vi "Multi_Run_Prog.vi"(0 "Command filename":path, 1 "Mode":T9(ring), 2 "Table":T6[](array[typedef]) {"Carrier_2 Q (l/min)" format="%#.2f"; "Row Duration (mins)" format="%#.1f"; "Row No" min=0; "Trace Gas Concentration (%)" min=0.0 format="%#_4f"; "Carrier_1 Q (l/min)" format="%#.4f"; "Start X" format="%#.2f"; "Start Y" format="%#.2f"; "Start Z" format="%#.2f"; "End X" format="%#.2f"; "End Y" format="%#.2f"; "End Z" format="%#.2f"; "Tunnel Speed" format="%#.2f"; "Averaging time (mins)" min=0.0 format="%#.2f"}, 3 "Work in Tunnel Coordinates?":T1) -> (17 "Status":T2)   [LabVIEW 2022 SP3]
uses:
  Anemometry Sub Vis/Gen Trav/Traverse_cluster.ctl
  Anemometry Sub Vis/Gen Trav/Spacing.ctl
  Anemometry Sub Vis/Controls/Multi_run_mode.ctl
  Anemometry Sub Vis/Gen Trav/Route mapping/Route_Display_Mode.ctl
  Anemometry Sub Vis/Controls/User_Specific_mode.ctl
  Anemometry Sub Vis/Controls/Multi_Run_Case.ctl
  Anemometry Sub Vis/Gen Trav/Multi_Run_Status.ctl
  Anemometry Sub Vis/Controls/Tunnel_Coordinates.ctl
  Anemometry Sub Vis/Controls/Post_Process.ctl
  ADAM Client/Sub VIs/ADAM Controls/Traverse_Level_State.ctl
  Anemometry Sub Vis/Controls/PP Raw data file cluster.ctl
  ADAM Client/Sub VIs/ADAM Controls/Tunnel_speed_mode.ctl
  Anemometry Sub Vis/Controls/Overhead.ctl
  ADAM Client/Sub VIs/ADAM Controls/Remember_value_mode.ctl
  Anemometry Sub Vis/Gen Trav/Trav_mode.ctl
  Anemometry Sub Vis/Controls/Home.ctl
  ADAM Client/Sub VIs/ADAM Controls/Quick_local_ADAM_Table.ctl
  ADAM Client/Sub VIs/ADAM Controls/Client_Source_Status.ctl
  ADAM Client/Sub VIs/ADAM Controls/Update_scan_value.ctl
  <vilib>/Utility/error.llb/Trim Whitespace One-Sided.vi
  Anemometry Sub Vis/Globals/Meas_global.vi
  Anemometry Sub Vis/Globals/Trav_pos_global.vi
  Anemometry Sub Vis/Globals/Preference_global.vi
  Anemometry Sub Vis/Globals/Extra_Commands_Global.vi
  Anemometry Sub Vis/Gen Trav/Route mapping/Route_mapping_global.vi
  ADAM Serial/Instrument drivers/Traverses/~subVIs/DriveConfigGlobal.vi
  Anemometry Sub Vis/Globals/Gas_management_global.vi
  <vilib>/Utility/config.llb/Write Key (Double).vi
  <vilib>/Utility/config.llb/NI_LVConfig.lvlib
panel:
  out "remainingTime":string
  out "Progress":i32(slide) scale=0.0..1.0
  out "PredictedEnd":timestamp format="%<%H:%M\n%a %d>T"
  out "StartTime":timestamp format="%<%H:%M\n%a %d>T"
  in  "Fast Plotting?":bool
  in  "Sort Single\nMeasurements":bool
  out "Last Row Run":i32
  in  "Stop after Repeats":bool
  out "Overhead Factor":dbl format="%.3f"
  out "Estimated Completion":string
  out "Max Tunnel Speed":dbl format="%.2f"
  out "Pause message":string
  in  "Pause":bool
  out "Non Starter":bool
  out "No of Rows":i32
  in  "Synchronization Start No":i32=1 min=1 max=100
  out "Case":T3
  out "Simulate/Run":T4
  in  "Display Mode":T5=enum."Display View on Crash"
  in  "stop":bool
  out "Current Row":i32
  # "X           Y          Z"
  # "Start"
  # "End"
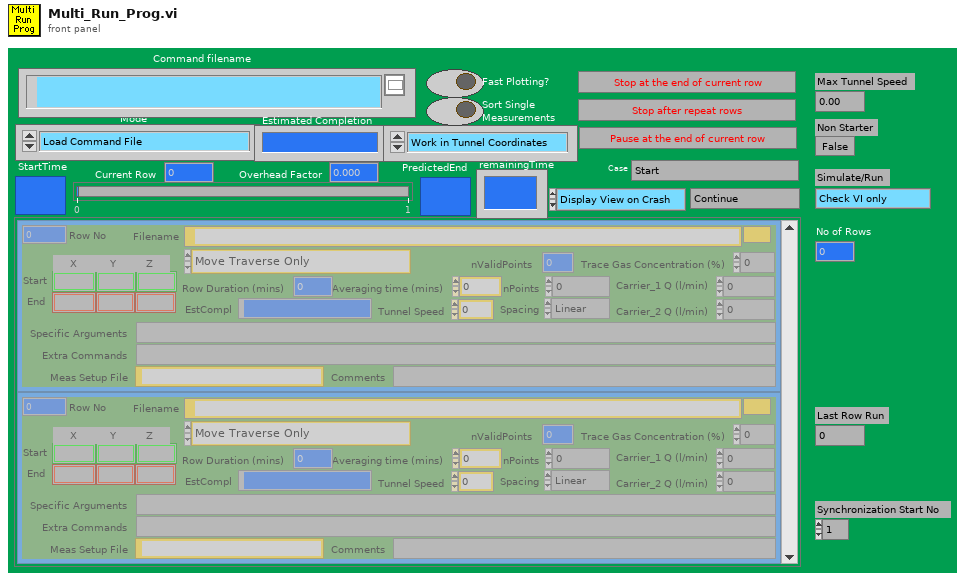
[diagram p1: front panel]
types:
  T1 = typedef "Tunnel_Coordinates.ctl" = enum16{"Work in Tunnel Coordinates", "Work in Model Coordinates"}
  T2 = typedef "Multi_Run_Status.ctl" = enum16{"Continue", "Continue with Error", "Jump to Next Point", "Jump to Next Row", "Jump To Fall Back", "Terminate Run"}
  T3 = typedef "Multi_Run_Case.ctl" = enum16{"Start", "Load Setup From File", "Has file been edited in Excel?", "Check Max Tunnel Speed", "Pre Check Row", "Check Rows", "Remove blank end rows", "Do results files already exist?", "More Multi Run Checks", "First Save Setup file", "Setup Route checking", "Initialise Measurement Prog", "Input Current Position", "Experimental setup control", "Check source flowrates", "Setup for running mode", "Skip Blank Rows", "Which row to execute next", "Evaluate IF Statement", "Perform Measurement Setup", "Set Measurement Conditions", "Execute Row", "Calculate Row TIme", "Update time estimate", "Pause Multi Run Program", "Do Another Row?", "Find Next Fall Back Row", "Shut down source etc", "Email results to users", "Save run efficiency", "Remove Skipped Commands", "Show jumped positions", "Save Setup to File", "End"}
  T4 = typedef "User_Specific_mode.ctl" = enum16{"Check VI only", "Run VI"}
  T5 = typedef "Route_Display_Mode.ctl" = enum16{"Display View Always", "Display View on Crash"}
  T6 = typedef "Traverse_cluster.ctl" = cluster{"Start X":sgl, "Start Y":sgl, "Start Z":sgl, "End X":sgl, "End Y":sgl, "End Z":sgl, "nPoints":i32, "Spacing":T7, "Filename":path, "Tunnel Speed":dbl, "Averaging time (mins)":dbl, "Extra Commands":string, "Carrier_1 Q (l/min)":dbl, "Carrier_2 Q (l/min)":dbl, "Trace Gas Concentration (%)":dbl, "Specific Arguments":string, "Comments":string, "Row No":i32, "Row Type Selector":T8, "EstCompl":string, "Row Duration (mins)":dbl, "nValidPoints":i32, "Meas Setup File":string}
  T7 = typedef "Spacing.ctl" = enum16{"Linear", "Log", "Gauss", "Specified", "N/A"}
  T8 = typedef "Multi_run_mode.ctl" = enum16{"Move Traverse Only", "Set Tunnel Speed Only", "Set Source Only", "Set Measurement Conditions", "Single Measurement", "Vertical Profile", "Lateral Profile", "Longitudinal Profile", "Multi-Axis Profile", "Explore Volume", "Auto Calibrate", "Meas Fast FID Bkgnd", "Check Beam Power", "Scanning Valve Measurement", "Run VI Named:", "Set ADAM Ch", "Wait (minutes)", "Send Message", "Synchronize With:", "Fall Back to this Row", "Turn Off Row Repeating", "Traverse 3D Volume", "Blank Row", "Jump to Fall Back Row"}
  T9 = enum16{"Load Command File", "Save Command File", "Check Multi Run Prog", "Check Multi Run Prog With Live Moves", "Run Multi Run Prog"}
  T10 = typedef "Post_Process.ctl" = enum16{"Take New Data", "Post Process Raw Data File"}
  T11 = typedef "PP Raw data file cluster.ctl" = cluster{"Raw Data File":path, "Results File":path}
  T12 = typedef "Traverse_Level_State.ctl" = enum16{"Running", "Complete"}
  T13 = enum32{"existing file", "new file", "new or existing file", "existing dir", "new dir", "new or existing dir", "existing file (use LLBs)", "new file (use LLBs)", "new or existing file (use LLBs)", "new or existing file or directory (use LLBs)"}
  T14 = typedef "Tunnel_speed_mode.ctl" = enum16{"Set Speed", "Set Speed then wait", "Is tunnel speed allowable?"}
  T15 = enum16{"All Channel Names", "Valid Channel Names"}
  T16 = typedef "Overhead.ctl" = enum16{"Update total times", "Read Current Overhead", "Re Scale totals to 3 hrs", "Initialise totals to 3hr"}
  T17 = typedef "Remember_value_mode.ctl" = enum16{"Read only", "Read and Write"}
  T18 = typedef "Home.ctl" = enum16{"Don't Home", "Home  +X", "Home  -X", "Home  +Y", "Home  -Y", "Home  +Z", "Home  -Z"}
  T19 = typedef "Trav_mode.ctl" = enum16{"Move traverse", "Read traverse position", "Teach Position"}
  T20 = typedef "Quick_local_ADAM_Table.ctl" = enum16{"Read Global", "Load Global From ADAM Table", "Write Global"}
  T21 = typedef "Client_Source_Status.ctl" = enum16{"Not Using", "Using", "Must Have"}
  T22 = typedef "Update_scan_value.ctl" = cluster{"Channel Name":string, "New Value":dbl, "!Auto_Off":bool}
  T23 = typedef "DriveProperties.ctl" = cluster{"Channel Name":string, "Vel. Default":sgl, "Acc. Default":sgl, "Vel. Max":sgl, "Vel. Min":sgl, "Acc. Max":sgl, "Acc. Min":sgl, "Pulses/unit":sgl, "Address":u8, "Pulse Offset":i32, "Pos Tolerance":sgl, "Pulses/rev":sgl, "Backlash/Eng units":sgl, "Current Pos":sgl, "Ch Status":enum16{"Active", "Offline", "Simulate"}, "Port Name":string, "Axis Transform mode":string, "Metadata Ch Name":string, "Type":T24, "De Power Motor":enum16{"TRUE", "FALSE"}, "ConfigString":string}
  T24 = typedef "Traverse Type.ctl" = enum16{"MCode", "Dynamixel"}
  T25 = typedef "GMU Gas Line Name.ctl" = enum16{"GMU1 Source", "GMU2 Source", "GMU2 Calib", "CPP GRC-A", "CPP GRC-B"}
  T26 = typedef "Status_Cluster.ctl" = cluster{"Status":T2, "Error Type":string, "Error Description":string}
  T27 = typedef "Server_Comms.ctl" = enum16{"Do Not Link To Server", "Server Link Healthy"}
  T28 = typedef "NI_LVConfig.lvlib/Config Data RefNum.ctl" = refnum<k1>
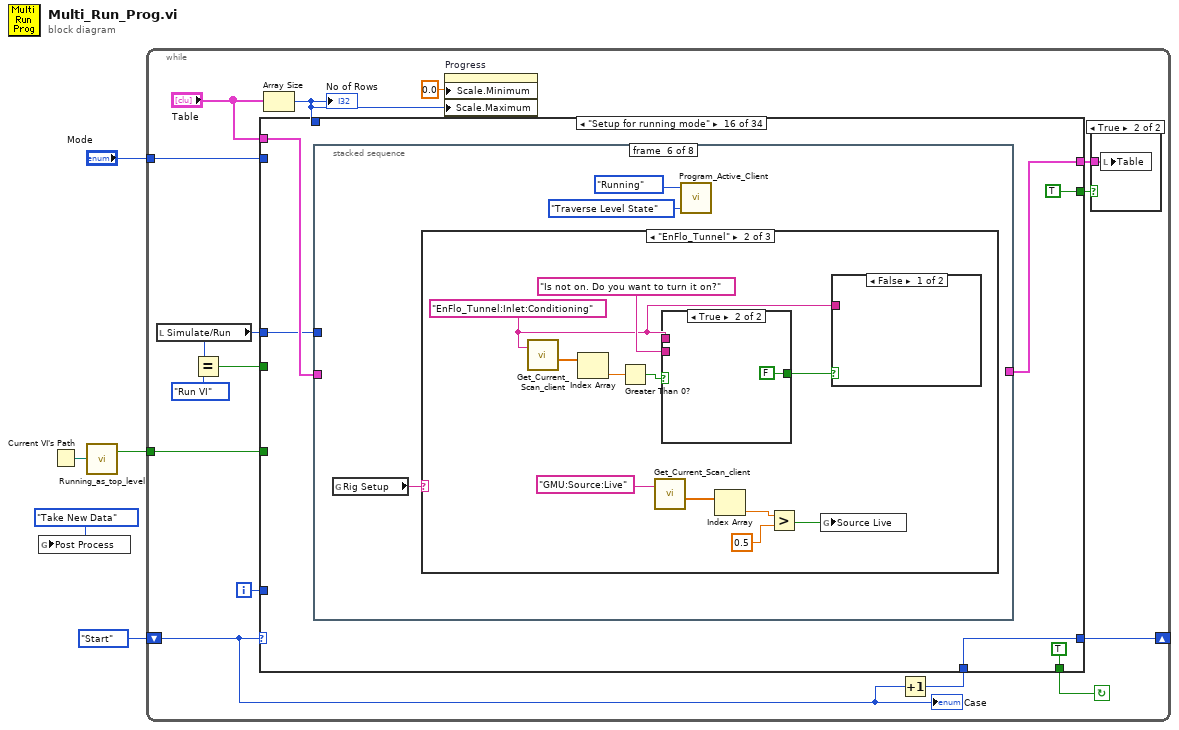
[diagram p0: block diagram]
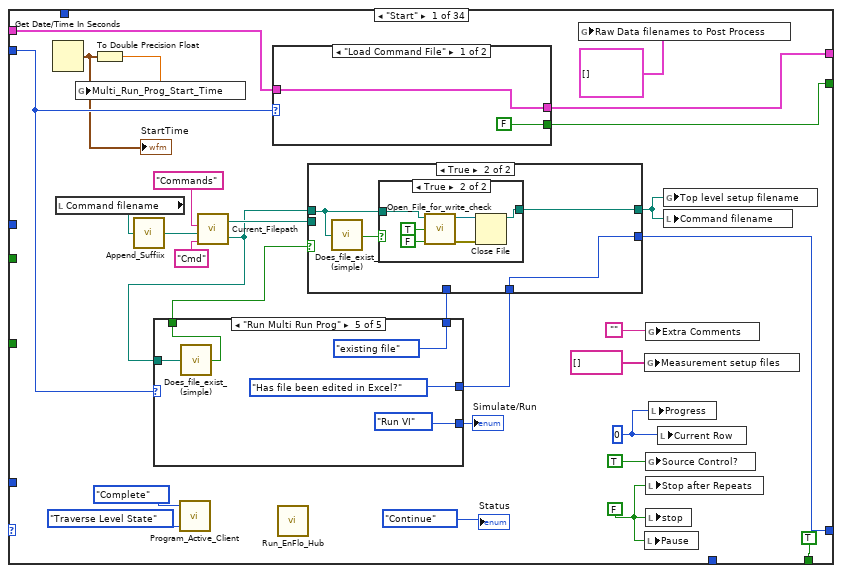
[diagram p3: hidden frame]
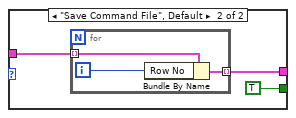
[diagram p4: hidden frame]
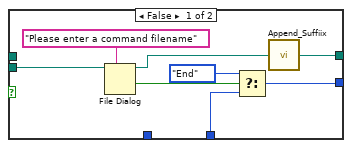
[diagram p5: hidden frame]
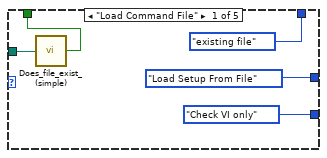
[diagram p7: hidden frame]
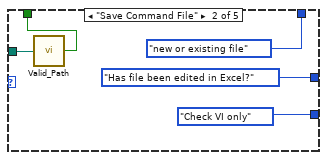
[diagram p8: hidden frame]
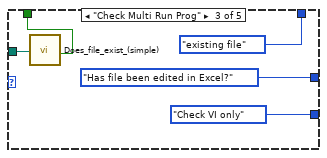
[diagram p9: hidden frame]
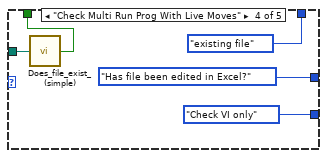
[diagram p10: hidden frame]
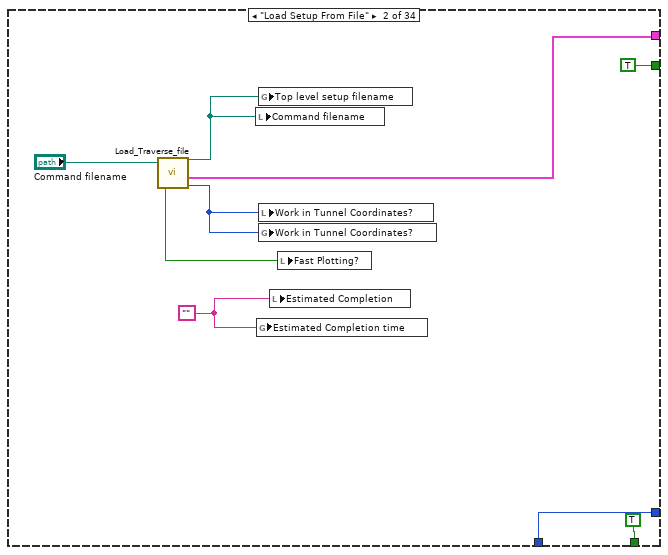
[diagram p11: hidden frame]
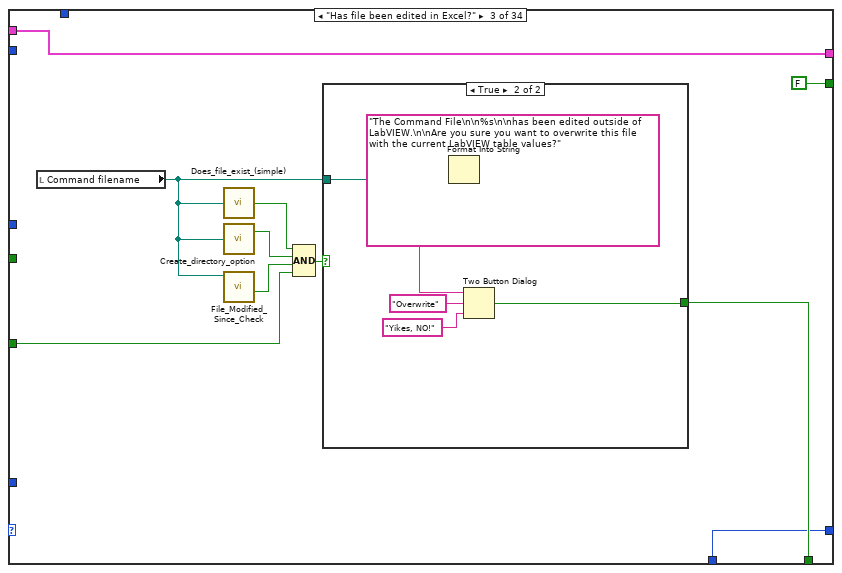
[diagram p12: hidden frame]
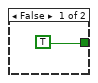
[diagram p13: hidden frame]
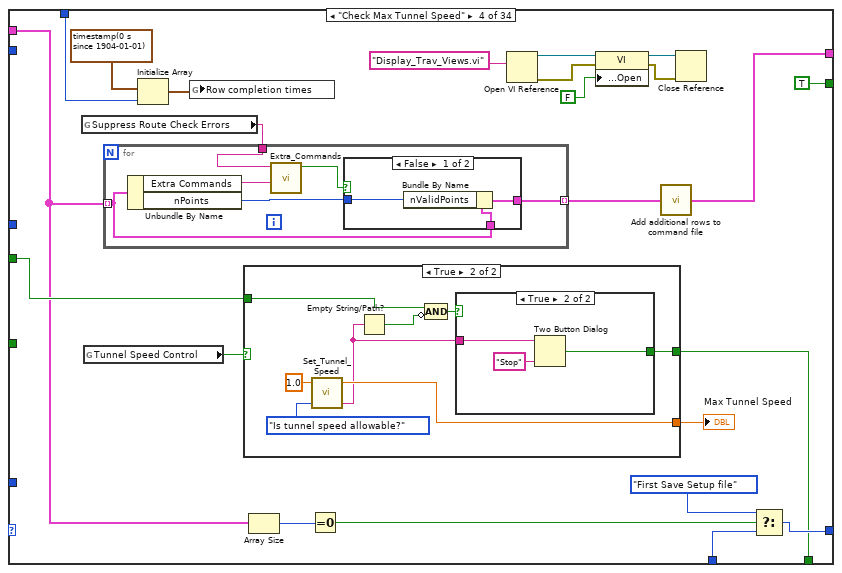
[diagram p14: hidden frame]
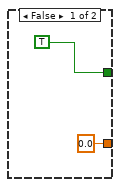
[diagram p16: hidden frame]
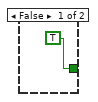
[diagram p17: hidden frame]
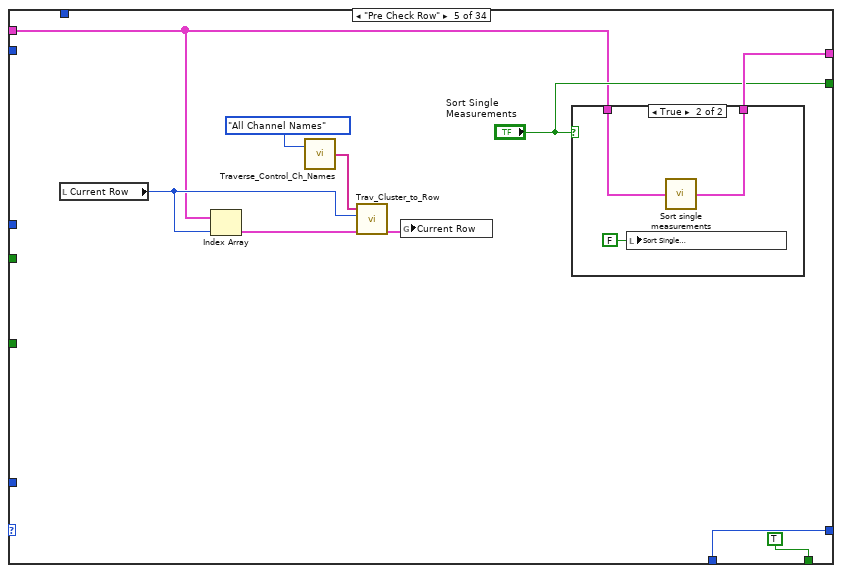
[diagram p18: hidden frame]
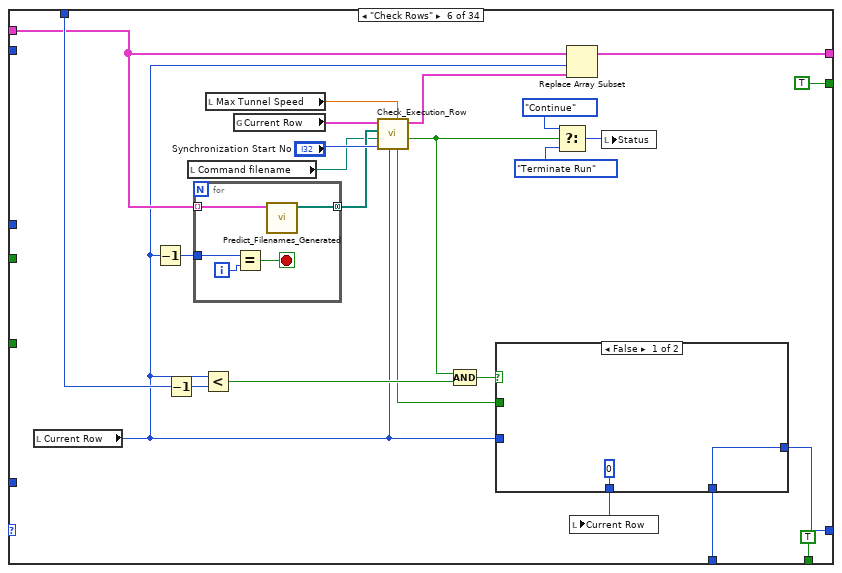
[diagram p20: hidden frame]
diagram:
  n1 = global write "Meas_global.vi" "Post Process"(Post_Process."Take New Data" ("Post Process")) -> ()
  n2 = Current VI's Path() -> (path=w2:path)
  n3 = call "Running_as_top_level.vi"("Vi path name"=w2) -> ("Top Level"=w1:bool)  [unwired: 1 out]
  n4 = while {
    shift-left: Multi_Run_Case."Start" ("Multi Run Case") -> [w17]
    shift-right: [w14] -> _
    tunnel: "Mode" -> [w20]
    tunnel: w1 -> [w9]
    i -> [w18]
    stop <- w8 continue-if-true
    n5 = local read "Simulate/Run"() -> (w11:T4)
    n6 = Equal?(x=w11, y=User_Specific_mode."Run VI" ("Simulate/Run")) -> (x = y?=w10:bool)
    n7 = Array Size(array="Table") -> (size(s)=w7:i32)
    "No of Rows" <- w7
    n8 = property on="Progress" class="Slide (strict)"("Scale.Minimum"=0.0 ("Scale.Range:Minimum"), "Scale.Maximum"=w7) -> ()  [unwired: 2 in, 2 out]
    n9 = Increment(x=w17) -> (x+1=w19:T3)
    n10 = case shown="\"Setup for running mode\"" w17 {
      tunnel: [TRUE TRUE w118 w134 TRUE TRUE TRUE TRUE TRUE TRUE TRUE ("Continue?") TRUE ("Continue?") TRUE TRUE TRUE TRUE ("Continue?") TRUE ("Continue?") TRUE ("Continue?") TRUE TRUE ("Continue?") TRUE TRUE TRUE TRUE TRUE TRUE TRUE TRUE TRUE TRUE TRUE TRUE TRUE FALSE] -> w8
      tunnel: w20 -> [w37 _ _ _ _ _ _ _ _ w539 _ _ _ _ _ _ _ _ _ _ _ _ _ _ _ _ _ _ _ _ _ _ w1456 _]
      tunnel: "Table" -> [w47 _ w115 w132 w175 w193 w232 w256 w413 w541 w564 w627 w645 w652 w660 w677 w766 w814 w935 w985 w998 w1089 w1128 w1160 w1203 w1247 w1289 w1334 w1366 w1414 w1425 w1443 w1475 w1525]
      tunnel: w11 -> [_ _ _ _ _ _ _ w255 _ _ _ _ _ _ w659 w676 _ w812 _ w982 w995 w1088 _ w1157 _ w1253 _ _ _ _ _ _ w1466 _]
      tunnel: w19 -> [_ w107 w117 w147 w183 w199 w243 w259 w412 w538 w567 w625 w646 w651 w664 w679 w768 w810 w940 w986 w1005 w1086 w1121 w1162 w1206 _ _ w1320 w1368 w1416 w1428 w1446 w1473 w1524]
      tunnel: w18 -> [_ _ _ _ _ _ _ _ _ _ _ _ _ _ _ _ _ _ _ _ _ _ _ _ w1204 _ _ _ _ _ _ _ _ _]
      tunnel: [w45 w107 w117 w146 w183 w198 w243 w259 w412 w534 w567 w624 w646 w651 w662 w679 w768 w811 w939 w986 w1006 w1086 w1121 w1162 w1207 w1242 w1296 w1329 w1368 w1416 w1428 w1446 w1473 w1524] -> w14
      tunnel: [w36 TRUE FALSE ("Rows Added ?") TRUE ("Rows Added ?") "Sort Single\nMeasurements" TRUE TRUE FALSE FALSE TRUE FALSE FALSE FALSE FALSE FALSE TRUE FALSE ("Rows Added ?") FALSE ("Rows Added ?") FALSE FALSE ("Rows Added ?") FALSE FALSE FALSE TRUE ("Rows Added ?") FALSE FALSE FALSE FALSE FALSE FALSE TRUE TRUE TRUE FALSE] -> w15
      tunnel: w7 -> [_ _ _ w141 _ w203 w234 _ _ _ _ _ _ _ _ _ w769 w813 _ _ _ _ _ w1156 _ w1245 w1291 _ _ _ _ _ w1452 _]
      tunnel: [w46 w108 w115 w129 w177 w206 w238 w256 w413 w542 w564 w627 w645 w652 w660 w675 w766 w815 w935 w985 w998 w1089 w1128 w1159 w1203 w1247 w1289 w1334 w1366 w1414 w1424 w1443 w1474 w1525] -> w13
      tunnel: w10 -> [_ _ _ w133 _ _ _ _ _ _ _ _ _ w649 w658 _ _ _ w929 _ _ _ w1120 _ _ _ _ _ _ _ _ _ _ _]
      tunnel: w9 -> [_ _ w114 _ _ _ _ w254 _ _ _ _ _ _ _ _ _ _ _ _ _ _ _ _ _ _ _ _ _ _ _ _ _ _]
      frame "Start" {
        w34 = FALSE ("Measurment setup Found?")
        w22 = 0 ("Currently on Row")
        n11 = Get Date/Time In Seconds() -> (seconds since 1Jan1904=w23:timestamp)
        "StartTime" <- w23
        n12 = local read "Command filename"() -> (w39:path)
        n13 = To Double Precision Float(number=w23) -> (double precision float=w25:dbl)
        n14 = global write "Trav_pos_global.vi" "Multi_Run_Prog_Start_Time"(w25) -> ()
        n15 = call "Append_Suffiix.vi"("Results file"=w39) -> ("appended path"=w30:path)
        n16 = call "Program_Active_Client.vi"("Mode"=enum16{"Program Active", "Traverse Level State"}."Traverse Level State", "Traverse level State"=Traverse_Level_State."Complete") -> ()  [unwired: 1 in, 3 out]
        n17 = call "Current_Filepath.vi"("Short_Name"="Cmd" ("Data Type"), "Filename in"=w30, "Data Type"="Commands") -> ("Filename Out"=w27:path, "Directory"=w29:path)  [unwired: 1 in]
        n18 = case shown="\"Run Multi Run Prog\"" w37 {
          tunnel: [User_Specific_mode."Check VI only" ("Simulate/Run") User_Specific_mode."Check VI only" ("Simulate/Run") User_Specific_mode."Check VI only" ("Simulate/Run") User_Specific_mode."Check VI only" ("Simulate/Run") User_Specific_mode."Run VI" ("Simulate/Run")] -> w48
          tunnel: [Multi_Run_Case."Load Setup From File" ("Multi Run Case") Multi_Run_Case."Has file been edited in Excel?" ("Multi Run Case") Multi_Run_Case."Has file been edited in Excel?" ("Multi Run Case") Multi_Run_Case."Has file been edited in Excel?" ("Multi Run Case") Multi_Run_Case."Has file been edited in Excel?" ("Multi Run Case")] -> w44
          tunnel: [T13."existing file" ("select mode (2)") T13."new or existing file" ("select mode (2)") T13."existing file" ("select mode (2)") T13."existing file" ("select mode (2)") T13."existing file" ("select mode (2)")] -> w35
          tunnel: w27 -> [w78 w83 w87 w93 w98]
          tunnel: [w77 w82 w88 w92 w97] -> w26
          frame "Load Command File" {
            n19 = call "Does_file_exist_(simple).vi"("Pathname"=w78) -> ("exists?"=w77:bool)
          }
          frame "Save Command File" {
            n20 = call "Valid_Path.vi"("Filename"=w83) -> ("Valid Path?"=w82:bool)
          }
          frame "Check Multi Run Prog" {
            n21 = call "Does_file_exist_(simple).vi"("Pathname"=w87) -> ("exists?"=w88:bool)
          }
          frame "Check Multi Run Prog With Live Moves" {
            n22 = call "Does_file_exist_(simple).vi"("Pathname"=w93) -> ("exists?"=w92:bool)
          }
          frame "Run Multi Run Prog" {
            n23 = call "Does_file_exist_(simple).vi"("Pathname"=w98) -> ("exists?"=w97:bool)
          }
        }
        "Simulate/Run" <- w48
        n24 = case shown="\"Load Command File\"" w37 {
          tunnel: w47 -> [w51 w54]
          tunnel: [w51 w53] -> w46
          tunnel: [FALSE TRUE] -> w36
          frame "Load Command File" {
          }
          frame "Save Command File", Default {
            n25 = for {
              tunnel: w54 -> [w57] mode=indexing
              tunnel: [w56] -> w53 mode=indexing
              i -> [w55]
              n26 = Bundle By Name(cluster=w57, "Row No"=w55) -> (w56:T6)
            }
          }
        }
        n27 = call "Run_EnFlo_Hub.vi"() -> ()  [unwired: 1 in, 7 out]
        n28 = case shown="True" w26 {
          tunnel: [w63 w69] -> w45
          tunnel: w44 -> [w64 w69]
          tunnel: w27 -> [_ w67]
          tunnel: [w62 w68] -> w38
          tunnel: w35 -> [_ _]
          tunnel: w29 -> [w58 _]
          frame False {
            n29 = File Dialog(7:"Please enter a command filename" ("prompt"), 11:w58) -> (1:w60:bool, 3:w61:path)  [unwired: 1 in, 6 out]
            n30 = Select(t=Multi_Run_Case."End" ("Multi Run Case"), s=w60, f=w64) -> (s? t:f=w63:T3)
            n31 = call "Append_Suffiix.vi"("Results file"=w61) -> ("appended path"=w62:path)
          }
          frame True {
            n32 = call "Does_file_exist_(simple).vi"("Pathname"=w67) -> ("exists?"=w66:bool)
            n33 = case shown="True" w66 {
              tunnel: [w70 w72] -> w68
              tunnel: w67 -> [w70 w71]
              frame False {
              }
              frame True {
                n34 = call "Open_File_for_write_check.vi"("advisory dialog? (display:T)"=FALSE, "append to file? (new file:F)"=TRUE, "file path"=w71) -> ("error out"=w74:errorcluster, "refnum"=w73:refnum<file>)  [unwired: 7 out]
                n35 = Close File(refnum=w73, error in=w74) -> (path=w72:path)  [unwired: 1 out]
              }
            }
          }
        }
        n36 = global write "Trav_pos_global.vi" "Raw Data filenames to Post Process"(T11[] [] ("Raw Data filenames to Post Process")) -> ()
        n37 = global write "Trav_pos_global.vi" "Measurement setup files"(string[] [] ("Measurement setup files")) -> ()
        n38 = local write "Pause"(w34) -> ()
        n39 = global write "Meas_global.vi" "Extra Comments"("") -> ()
        n40 = global write "Trav_pos_global.vi" "Source Control?"(TRUE ("Source Control?")) -> ()
        n41 = local write "Stop after Repeats"(w34) -> ()
        n42 = local write "stop"(w34) -> ()
        n43 = local write "Progress"(w22) -> ()
        n44 = local write "Current Row"(w22) -> ()
        n45 = global write "Trav_pos_global.vi" "Top level setup filename"(w38) -> ()
        n46 = local write "Command filename"(w38) -> ()
        "Status" <- Multi_Run_Status."Continue" ("Status")
      }
      frame "Load Setup From File" {
        w103 = ""
        n47 = call "Load_Traverse_file.vi"("Setup filename"="Command filename") -> ("Fast Plotting?"=w102:bool, "Setup filename Out"=w105:path, "Table"=w108:T6[], "Work in Tunnel Coordinates?"=w104:T1)  [unwired: 2 out]
        n48 = local write "Command filename"(w105) -> ()
        n49 = global write "Trav_pos_global.vi" "Estimated Completion time"(w103) -> ()
        n50 = global write "Trav_pos_global.vi" "Top level setup filename"(w105) -> ()
        n51 = local write "Work in Tunnel Coordinates?"(w104) -> ()
        n52 = global write "Trav_pos_global.vi" "Work in Tunnel Coordinates?"(w104) -> ()
        n53 = local write "Estimated Completion"(w103) -> ()
        n54 = local write "Fast Plotting?"(w102) -> ()
      }
      frame "Has file been edited in Excel?" {
        n55 = local read "Command filename"() -> (w112:path)
        n56 = call "Does_file_exist_(simple).vi"("Pathname"=w112) -> ("exists?"=w113:bool)
        n57 = call "Create_directory_option.vi"("Filename"=w112) -> ("Path is to existing File"=w119:bool)  [unwired: 1 out]
        n58 = call "File_Modified_Since_Check.vi"("File Path"=w112) -> ("modifiedSinceRead"=w111:bool)  [unwired: 7 in, 1 out]
        n59 = Compound Arithmetic op=AND(w113, w119, w111, w114) -> (w120:bool)
        n60 = case shown="True" w120 {
          tunnel: w112 -> [_ w127]
          tunnel: [TRUE ("T button?") w122] -> w118
          frame False {
          }
          frame True {
            n61 = Format Into String(format string="The Command File\n\n%s\n\nhas been edited outside of LabVIEW.\n\nAre you sure you want to overwrite this file with the current LabVIEW table values?" ("Format String"), w127) -> (resulting string=w125:string)  [unwired: 2 in, 1 out]
            n62 = Two Button Dialog(message=w125, 1:"Yikes, NO!" ("F button name (\"Cancel\")"), 2:"Overwrite" ("T button name (\"OK\")")) -> (T button?=w122:bool)
          }
        }
      }
      frame "Check Max Tunnel Speed" {
        n63 = global read "Extra_Commands_Global.vi" "Suppress Route Check Errors"() -> (w128:string)
        n64 = global read "Preference_global.vi" "Tunnel Speed Control"() -> (w131:bool)
        n65 = for {
          tunnel: w132 -> [w155] mode=indexing
          tunnel: [w154] -> w130 mode=indexing
          tunnel: w128 -> [w152]
          n66 = Unbundle By Name(w155) -> ("Extra Commands"=w153:string, "nPoints"=w156:i32)
          n67 = call "Extra_Commands.vi"("String to Search"=w153, "Command"=w152) -> ("Command Found"=w151:bool)  [unwired: 1 in, 4 out]
          n68 = case shown="False" w151 {
            tunnel: w156 -> [w159 _]
            tunnel: w155 -> [w158 w160]
            tunnel: [w157 w160] -> w154
            frame False {
              n69 = Bundle By Name(cluster=w158, "nValidPoints"=w159) -> (w157:T6)
            }
            frame True {
            }
          }
        }
        n70 = Initialize Array(timestamp(0 s since 1904-01-01) ("seconds since 1Jan1904"), w141) -> (w142:timestamp[])
        n71 = global write "Trav_pos_global.vi" "Row completion times"(w142) -> ()
        n72 = case shown="True" w131 {
          tunnel: [0.0 ("Max allowable Tunnel Velocity") w169] -> w150
          tunnel: [TRUE w166] -> w134
          tunnel: w133 -> [_ w164]
          frame False {
          }
          frame True {
            n73 = call "Set_Tunnel_Speed.vi"("Mode"=Tunnel_speed_mode."Is tunnel speed allowable?", "Tunnel Velocity m/s"=1.0) -> ("Error String"=w167:string, "Max allowable Tunnel Velocity"=w169:dbl)  [unwired: 1 in, 1 out]
            n74 = Empty String/Path?(string/path=w167) -> (empty?=w165:bool)
            n75 = Compound Arithmetic op=AND(w164, invert w165) -> (w163:bool)
            n76 = case shown="True" w163 {
              tunnel: w167 -> [_ w174]
              tunnel: [TRUE ("T button?") w172] -> w166
              frame False {
              }
              frame True {
                n77 = Two Button Dialog(message=w174, 1:"Stop" ("F button name (\"Cancel\")")) -> (T button?=w172:bool)  [unwired: 1 in]
              }
            }
          }
        }
        "Max Tunnel Speed" <- w150
        n78 = Array Size(array=w132) -> (size(s)=w148:i32)
        n79 = Equal To 0?(x=w148) -> (x = 0?=w145:bool)
        n80 = Open VI Reference(vi path="Display_Trav_Views.vi" ("VI path")) -> (vi reference=w140:refnum<vi>, error out=w139:errorcluster)  [unwired: 1 in, 4 out]
        n81 = property class="VI"(reference=w140, error in=w139, "Front Panel Window:Open"=FALSE) -> (reference out=w137:refnum<vi>, error out=w136:errorcluster)
        n82 = call "Add additional rows to command file.vi"("Table In"=w130) -> ("Table Out"=w129:T6[])
        n83 = Close Reference(reference=w137, error in (no error)=w136) -> ()  [unwired: 1 out]
        n84 = Select(t=Multi_Run_Case."First Save Setup file" ("Multi Run Case"), s=w145, f=w147) -> (s? t:f=w146:T3)
      }
      frame "Pre Check Row" {
        n85 = local read "Current Row"() -> (w180:i32)
        n86 = Index Array(array=w175, index=w180) -> (element=w181:T6)
        n87 = call "Traverse_Control_Ch_Names.vi"("Mode"=T15."All Channel Names") -> ("Channel names"=w178:string[])  [unwired: 1 in]
        n88 = call "Trav_Cluster_to_Row.vi"("Traverse line in"=w181, "Row Number"=w180, "Channel names"=w178) -> ("Traverse line Out"=w182:T6)  [unwired: 4 out]
        n89 = global write "Trav_pos_global.vi" "Current Row"(w182) -> ()
        n90 = case shown="True" "Sort Single\nMeasurements" {
          tunnel: w175 -> [w185 w188]
          tunnel: [w185 w187] -> w177
          frame False {
          }
          frame True {
            n91 = local write "Sort Single\nMeasurements"(FALSE ("Sort Single\nMeasurements")) -> ()
            n92 = call "Sort single measurements.vi"("Table In"=w188) -> ("Table Out"=w187:T6[])
          }
        }
      }
      frame "Check Rows" {
        n93 = local read "Current Row"() -> (w192:i32)
        n94 = Decrement(x=w192) -> (x-1=w191:i32)
        n95 = Decrement(x=w203) -> (x-1=w196:i32)
        n96 = local read "Command filename"() -> (w189:path)
        n97 = for {
          tunnel: w193 -> [w217] mode=indexing
          tunnel: w191 -> [w215]
          tunnel: [w213] -> w190 mode=concatenating
          i -> [w216]
          stop <- w214 stop-if-true
          n98 = Equal?(x=w215, y=w216) -> (x = y?=w214:bool)
          n99 = call "Predict_Filenames_Generated.vi"("Traverse line"=w217) -> ("Filename"=w213:path[])  [unwired: 10 in]
        }
        n100 = Less?(x=w192, y=w196) -> (x < y?=w202:bool)
        n101 = local read "Max Tunnel Speed"() -> (w205:dbl)
        n102 = global read "Trav_pos_global.vi" "Current Row"() -> (w194:T6)
        n103 = call "Check_Execution_Row.vi"("Execution Row"=w194, "Earlier Filenames"=w190, "multirunFilepath"=w189, "Synchronization Start No"="Synchronization Start No", "Row Index"=w192, "Max Tunnel Speed"=w205) -> ("Edited Row"=w195:bool, "Execution Row Out"=w197:T6, "Continue?"=w204:bool)  [unwired: 2 out]
        n104 = Compound Arithmetic op=AND(w204, w202) -> (w201:bool)
        n105 = case shown="False" w201 {
          tunnel: [0 w221] -> w200
          tunnel: w192 -> [_ w225]
          tunnel: w199 -> [w219 _]
          tunnel: [w219 Multi_Run_Case."Pre Check Row" ("Multi Run Case")] -> w198
          tunnel: w195 -> [_ w223]
          frame False {
          }
          frame True {
            n106 = Increment(x=w225) -> (x+1=w222:i32)
            n107 = Select(t=0, s=w223, f=w222) -> (s? t:f=w221:i32)
          }
        }
        n108 = Select(t=Multi_Run_Status."Continue" ("Status"), s=w204, f=Multi_Run_Status."Terminate Run" ("Status")) -> (s? t:f=w210:T2)
        n109 = Replace Array Subset(array=w193, new element=w197, index=w192) -> (w206:T6[])
        n110 = local write "Current Row"(w200) -> ()
        n111 = local write "Status"(w210) -> ()
      }
      frame "Remove blank end rows" {
        n112 = call "Calc_Remaining_Time.vi"("Table In"=w232, "Currently on Row"=-1 ("Start Index")) -> ("Table Out"=w233:T6[], "noWaitCompletion"=w227:timestamp, "remainingTime"=→"remainingTime":string)  [unwired: 1 out]
        n113 = Reverse 1D Array(array=w233) -> (reversed array=w242:T6[])
        n114 = while {
          tunnel: [w245] -> w240
          tunnel: w234 -> [w249]
          tunnel: w242 -> [w253] mode=indexing
          i -> [w245]
          stop <- w246 continue-if-true
          n115 = Unbundle By Name(w253) -> ("Row Type Selector"=w251:T8)
          n116 = Increment(x=w245) -> (x+1=w250:i32)
          n117 = Greater?(x=w249, y=w250) -> (0:w248:bool)
          n118 = Equal?(x=Multi_run_mode."Blank Row" ("Row Type Selector"), y=w251) -> (x = y?=w247:bool)
          n119 = And(x=w247, y=w248) -> (x .and. y?=w246:bool)
        }
        n120 = Decrement(x=w234) -> (x-1=w231:i32)
        n121 = local write "PredictedEnd"(w227) -> ()
        n122 = Index Array(array=w233, index=w231) -> (element=w230:T6)
        n123 = Subtract(x=w234, y=w240) -> (x-y=w239:i32)
        n124 = Unbundle By Name(w230) -> ("EstCompl"=w228:string)
        n125 = call "Overhead_Factor.vi"("Mode"=Overhead."Read Current Overhead") -> ("Current Overhead Factor"=w235:dbl)  [unwired: 3 in]
        n126 = local write "Overhead Factor"(w235) -> ()
        n127 = global write "Trav_pos_global.vi" "Estimated Completion time"(w228) -> ()
        n128 = local write "Estimated Completion"(w228) -> ()
        n129 = Array Subset(array=w233, index=0 ("Array Index"), length=w239) -> (w238:T6[])
      }
      frame "Do results files already exist?" {
        n130 = for {
          tunnel: w256 -> [w269] mode=indexing
          shift-right: [w265] -> _
          shift-left: path[] [] -> [w266]
          tunnel: w255 -> [w263]
          tunnel: w254 -> [w261]
          n131 = Unbundle By Name(w269) -> ("Specific Arguments"=w262:string, "Row Type Selector"=w268:T8, "Filename"=w267:path)
          n132 = while {
            shift-left: w266 -> [w278]
            shift-right: [w277] -> w265
            tunnel: w267 -> [w279]
            tunnel: w268 -> [w283]
            shift-left: 0 -> [w284]
            shift-right: [w280] -> _
            tunnel: w263 -> [w274]
            shift-right: [w273] -> _
            shift-left: _ -> [w272]
            tunnel: w262 -> [w271]
            tunnel: w261 -> [w270]
            stop <- w282 continue-if-true
            n133 = Increment(x=w284) -> (x+1=w281:i32)
            n134 = case shown="0, Default" w284 {
              tunnel: w283 -> [w294 _ _ _ _ _ _ _ _ _ _ _]
              tunnel: [w289 w316 w321 w328 w333 TRUE ("exists?") TRUE ("exists?") FALSE ("exists?") FALSE ("exists?") TRUE ("true") w390 w403] -> w282
              tunnel: w281 -> [w296 w319 w324 w327 w334 w339 w350 w361 w372 w376 w388 _]
              tunnel: [w296 w319 w324 w327 w334 w337 w349 w361 w372 w377 w388 w402] -> w280
              tunnel: [w295 w318 w323 w326 w331 w347 w358 w363 w365 w374 w392 w408] -> w277
              tunnel: w278 -> [w295 w318 w323 w326 w332 w347 w358 w363 w365 w374 w392 w408]
              tunnel: w279 -> [w288 _ _ _ _ _ _ _ _ _ _ _]
              tunnel: 7 -> [_ _ _ _ _ _ _ _ _ w375 _ w402]
              tunnel: 9 -> [_ _ _ _ _ w338 _ _ _ _ _ _]
              tunnel: w274 -> [_ _ _ _ _ _ _ _ _ _ w391 _]
              tunnel: [w287 w315 w320 w325 w330 w335 w348 w359 w364 w373 w389 w401] -> w273
              tunnel: w272 -> [_ w315 w320 w325 w330 w335 w348 w359 w364 w373 w389 w401]
              tunnel: w271 -> [w286 _ _ _ _ _ _ _ _ _ _ _]
              tunnel: w270 -> [w285 _ _ _ _ _ _ _ _ _ _ _]
              frame 0, Default {
                n135 = case shown="\"Run VI Named:\"" w294 {
                  tunnel: [TRUE w307 FALSE FALSE] -> w291
                  tunnel: w288 -> [w297 w306 w311 w313]
                  tunnel: w286 -> [_ w304 _ _]
                  tunnel: [w297 w306 w311 w313] -> w287
                  frame "Move Traverse Only", Default {
                  }
                  frame "Run VI Named:" {
                    n136 = Match Pattern(string=w304, regular expression=";") -> (before substring=w303:string)  [unwired: 4 out]
                    n137 = call <vilib>:"Trim Whitespace.vi"("string"=w303) -> ("trimmed string"=w301:string)  [unwired: 1 in]
                    n138 = Equal?(x=w301, y="Pressure_Tapped_Cube.vi") -> (x = y?=w308:bool)
                    n139 = Equal?(x=w301, y="Take_Data_on_the_Move.vi") -> (x = y?=w302:bool)
                    n140 = Equal?(x=w301, y="Capture_Flow_Vis.vi") -> (x = y?=w299:bool)
                    n141 = Compound Arithmetic op=OR(w308, w302, w299) -> (w307:bool)
                  }
                  frame "Auto Calibrate" {
                  }
                  frame "Send Message" {
                  }
                }
                n142 = local read "Status"() -> (w292:T2)
                n143 = Not Equal?(x=Multi_Run_Status."Terminate Run" ("Status"), y=w292) -> (x != y?=w290:bool)
                n144 = Compound Arithmetic op=AND(w291, w290, w285) -> (w289:bool)
              }
              frame 1 {
                n145 = Not Equal?(x=path "", y=w315) -> (x != y?=w316:bool)
              }
              frame 2 {
                n146 = Not Equal?(x=w320, y=path "") -> (x != y?=w321:bool)
              }
              frame 3 {
                n147 = Search 1D Array(1D array=w326, element=w325) -> (index of element=w329:i32)  [unwired: 1 out]
                n148 = Less Than 0?(x=w329) -> (x < 0?=w328:bool)
              }
              frame 4 {
                n149 = Build Array (concatenate)(w332, w330) -> (w331:path[])
                n150 = call "Does_file_exist_(simple).vi"("Pathname"=w330) -> ("exists?"=w333:bool)
              }
              frame 5 {
                n151 = Path To String(path=w335) -> (string=w346:string)
                n152 = global read "Meas_global.vi" "Start Time of experiment"() -> (w341:dbl)
                n153 = Concatenate Strings(w346, "Append" ("Substring")) -> (w344:string)
                n154 = call "Remember_value.vi"("Mode"=Remember_value_mode."Read only", "Ch name"=w344) -> ("Output Value"=w342:dbl)  [unwired: 1 in]
                n155 = Not Equal?(x=w341, y=w342) -> (x != y?=w340:bool)
                n156 = Select(t=w339, s=w340, f=w338) -> (s? t:f=w337:i32)
              }
              frame 6 {
                n157 = Increment(x=w350) -> (x+1=w351:i32)
                n158 = Format Into String(format string="The results filename \"%s\" already exists.\nDo you wish to append to this file during the run?" ("Format String"), w348) -> (resulting string=w355:string)  [unwired: 2 in, 1 out]
                n159 = Two Button Dialog(message=w355, 1:"Abort Run" ("F button name (\"Cancel\")"), 2:"Append" ("T button name (\"OK\")")) -> (T button?=w352:bool)
                n160 = Select(t=w351, s=w352, f=w350) -> (s? t:f=w349:i32)
              }
              frame 7 {
                n161 = local write "Status"(Multi_Run_Status."Terminate Run" ("Status")) -> ()
              }
              frame 8 {
                n162 = Path To String(path=w364) -> (string=w371:string)
                n163 = Concatenate Strings(w371, "Append" ("Substring")) -> (w369:string)
                n164 = global read "Meas_global.vi" "Start Time of experiment"() -> (w366:dbl)
                n165 = call "Remember_value.vi"("Mode"=Remember_value_mode."Read and Write", "Input Value"=w366, "Ch name"=w369) -> ()  [unwired: 1 out]
              }
              frame 9 {
                n166 = call "Read_File_Simple.vi"("Filename"=w373) -> ("string"=w380:string)  [unwired: 2 in, 7 out]
                n167 = call "Is_it_a_Results_File.vi"("character string"=w380) -> ("Results File?"=w379:bool)  [unwired: 2 out]
                n168 = case shown="False" w379 {
                  tunnel: w373 -> [w383 _]
                  tunnel: [w381 w387] -> w377
                  tunnel: w376 -> [_ w387]
                  tunnel: w375 -> [w381 _]
                  frame False {
                    n169 = Path To String(path=w383) -> (string=w385:string)
                    n170 = Format Into String(format string="The File %s is not in the correct Results file format.\nCheck that it is tab delimited rather than excel format, or choose another file." ("Format String"), w385) -> (resulting string=w382:string)  [unwired: 2 in, 1 out]
                    n171 = One Button Dialog(message=w382, button name ("OK")="Stop") -> ()  [unwired: 1 out]
                  }
                  frame True {
                  }
                }
              }
              frame 10 {
                n172 = case shown="\"Check VI only\", Default" w391 {
                  tunnel: w389 -> [_ w400]
                  tunnel: [FALSE ("exists?") w394] -> w390
                  frame "Check VI only", Default {
                  }
                  frame "Run VI" {
                    n173 = call "Open_File_for_write.vi"("append to file? (new file:F)"=TRUE, "file path"=w400) -> ("error out"=w398:errorcluster, "refnum"=w399:refnum<file>)  [unwired: 1 in, 7 out]
                    n174 = Unbundle By Name(w398) -> ("code"=w397:i32)
                    n175 = Close File(refnum=w399, error in=w398) -> ()  [unwired: 2 out]
                    n176 = Equal?(x=10 ("code"), y=w397) -> (x = y?=w394:bool)
                  }
                }
              }
              frame 11 {
                n177 = Path To String(path=w401) -> (string=w406:string)
                n178 = Format Into String(format string="The File %s is already open in another application." ("Format String"), w406) -> (resulting string=w405:string)  [unwired: 2 in, 1 out]
                n179 = One Button Dialog(message=w405, button name ("OK")="Stop") -> (true=w403:bool)
              }
            }
          }
        }
      }
      frame "More Multi Run Checks" {
        n180 = global read "Preference_global.vi" "Rig Setup"() -> (w411:string)
        n181 = Equal?(x=w411, y="EnFlo_Tunnel") -> (x = y?=w409:bool)
        n182 = stacked-sequence {
          seq-local: [_ w434 _ _ _ _] -> [_ _ w447 _ _ _]
          seq-local: [_ _ _ _ w475 _] -> [_ _ _ _ _ w502]
          seq-local: [_ _ w444 _ _ _] -> [_ _ _ w463 _ _]
          tunnel: w413 -> [w418 w435 _ _ w476 _]
          tunnel: w409 -> [_ _ _ w465 w477 _]
          frame #0 {
            n183 = for {
              tunnel: w418 -> [w425] mode=indexing
              tunnel: [w423] -> w417 mode=indexing
              n184 = Unbundle By Name(w425) -> ("Specific Arguments"=w424:string, "Carrier_1 Q (l/min)"=w421:dbl, "Carrier_2 Q (l/min)"=w420:dbl, "Row Type Selector"=w422:T8)
              n185 = Add(x=w421, y=w420) -> (x+y=w419:dbl)
              n186 = case shown="\"Auto Calibrate\"" w422 {
                tunnel: w419 -> [w427 _]
                tunnel: w424 -> [_ w429]
                tunnel: [w426 w428] -> w423
                frame Default {
                  n187 = Greater Than 0?(x=w427) -> (x > 0?=w426:bool)
                }
                frame "Auto Calibrate" {
                  n188 = call "Get_array_values_fr_String.vi"("String Value"=w429) -> ("String array"=w432:string[])  [unwired: 1 out]
                  n189 = Index Array(array=w432, index=0 ("Index")) -> (element=w431:string)
                  n190 = Equal?(x=w431, y="Concentration") -> (x = y?=w428:bool)
                }
              }
            }
            n191 = Or Array Elements(Boolean array=w417) -> (logical OR=w416:bool)
            n192 = global write "Trav_pos_global.vi" "Source Control?"(w416) -> ()
          }
          frame #1 {
            n193 = global read "Trav_pos_global.vi" "Source Control?"() -> (w436:bool)
            n194 = case shown="True" w436 {
              tunnel: w435 -> [_ w440]
              tunnel: [FALSE w438] -> w434
              frame False {
              }
              frame True {
                n195 = for {
                  tunnel: w440 -> [w443] mode=indexing
                  tunnel: [w441] -> w439 mode=indexing
                  n196 = Unbundle By Name(w443) -> ("Trace Gas Concentration (%)"=w442:dbl)
                  n197 = Greater Than 0?(x=w442) -> (x > 0?=w441:bool)
                }
                n198 = Or Array Elements(Boolean array=w439) -> (logical OR=w438:bool)
              }
            }
          }
          frame #2 {
            n199 = global read "Preference_global.vi" "Site Specific String (Blank if Surrey)"() -> (w446:string)
            n200 = Empty String/Path?(string/path=w446) -> (empty?=w445:bool)
            n201 = Compound Arithmetic op=AND(w445, w447) -> (w444:bool)
            n202 = case shown="True" w444 {
              tunnel: [TRUE ("T button?") w453] -> _
              frame False {
              }
              frame True {
                w449 = "EnFlo_Tunnel:Gas Solenoid:Status"
                n203 = call "Get_Current_Scan_client.vi"("singleChannel"=w449) -> ("Numerical Values"=w455:dbl[])  [unwired: 1 in, 3 out]
                n204 = Index Array(array=w455, index=0) -> (element=w452:dbl)
                n205 = Greater?(x=w452, y=0.5) -> (0:w450:bool)
                n206 = case shown="False" w450 {
                  tunnel: w449 -> [w461 _]
                  tunnel: [w457 TRUE ("T button?")] -> w453
                  frame False {
                    n207 = Format Into String(format string="The \"%s\" ADAM channel is showing that the blue gas button is not on.", w461) -> (resulting string=w456:string)  [unwired: 2 in, 1 out]
                    n208 = Two Button Dialog(message=w456, 1:"Stop" ("F button name (\"Cancel\")"), 2:"Continue" ("T button name (\"OK\")")) -> (T button?=w457:bool)
                  }
                  frame True {
                  }
                }
              }
            }
          }
          frame #3 {
            n209 = Or(x=w463, y=w465) -> (x .or. y?=w464:bool)
            n210 = case shown="True" w464 {
              frame False {
              }
              frame True {
                w466 = "EnFlo_Tunnel:Safety_Loop:Status"
                n211 = call "Get_Current_Scan_client.vi"("singleChannel"=w466) -> ("Numerical Values"=w471:dbl[])  [unwired: 1 in, 3 out]
                n212 = Index Array(array=w471, index=0) -> (element=w469:dbl)
                n213 = Greater?(x=w469, y=0.5) -> (0:w467:bool)
                n214 = case shown="False" w467 {
                  tunnel: w466 -> [w474 _]
                  frame False {
                    n215 = Format Into String(format string="The \"%s\" ADAM channel is showing that the General Safety Loop is not on.", w474) -> (resulting string=w472:string)  [unwired: 2 in, 1 out]
                    n216 = One Button Dialog(message=w472) -> ()  [unwired: 1 in, 1 out]
                  }
                  frame True {
                  }
                }
              }
            }
          }
          frame #4 {
            n217 = case shown="True" w477 {
              tunnel: w476 -> [_ w483]
              tunnel: [FALSE w479] -> w475
              frame False {
              }
              frame True {
                w481 = "EnFlo_Tunnel:Setpoint:"
                n218 = String Length(string=w481) -> (length=w482:i32)
                n219 = for {
                  tunnel: w483 -> [w488] mode=indexing
                  tunnel: w482 -> [w486]
                  tunnel: w481 -> [w485]
                  tunnel: [w484] -> w480 mode=indexing
                  n220 = Unbundle By Name(w488) -> ("Row Type Selector"=w487:T8, "Specific Arguments"=w489:string)
                  n221 = case shown="\"Set ADAM Ch\"" w487 {
                    tunnel: w489 -> [_ w496]
                    tunnel: w486 -> [_ w495]
                    tunnel: w485 -> [_ w493]
                    tunnel: [FALSE w491] -> w484
                    frame "Move Traverse Only", Default {
                    }
                    frame "Set ADAM Ch" {
                      n222 = call "Get_array_values_fr_String.vi"("String Value"=w496) -> ("String array"=w494:string[])  [unwired: 1 out]
                      n223 = for {
                        tunnel: w495 -> [w501]
                        tunnel: w494 -> [w500] mode=indexing
                        tunnel: w493 -> [w498]
                        tunnel: [w497] -> w492 mode=indexing
                        n224 = String Subset(string=w500, length (rest)=w501) -> (substring=w499:string)  [unwired: 1 in]
                        n225 = Equal?(x=w499, y=w498) -> (x = y?=w497:bool)
                      }
                      n226 = Or Array Elements(Boolean array=w492) -> (logical OR=w491:bool)
                    }
                  }
                }
                n227 = Or Array Elements(Boolean array=w480) -> (logical OR=w479:bool)
              }
            }
          }
          frame #5 {
            w503 = "Uni:Chilled Water:Temp"
            w504 = "EnFlo_Tunnel:Heater:Enable"
            n228 = Build Array(w504, w503) -> (w508:string[])
            n229 = call "Get_Current_Scan_client.vi"("multipleChannels"=w508) -> ("Numerical Values"=w509:dbl[])  [unwired: 1 in, 3 out]
            n230 = Index Array(array=w509) -> (element #1=w510:dbl, element #2=w506:dbl)  [unwired: 2 in]
            n231 = Greater?(x=w510, y=0.5) -> (0:w507:bool)
            n232 = case shown="True" w502 {
              tunnel: w507 -> [_ w514]
              tunnel: w504 -> [_ w513]
              tunnel: w506 -> [_ w512]
              tunnel: w503 -> [_ w511]
              frame False {
              }
              frame True {
                n233 = stacked-sequence {
                  tunnel: w514 -> [w516 _]
                  tunnel: w513 -> [w515 w524]
                  tunnel: w512 -> [_ w520]
                  tunnel: w511 -> [_ w521]
                  frame #0 {
                    n234 = case shown="False" w516 {
                      tunnel: w515 -> [w519 _]
                      frame False {
                        n235 = Format Into String(format string="The \"%s\" have not been enabled but the run is changing heater setpoints.", w519) -> (resulting string=w517:string)  [unwired: 2 in, 1 out]
                        n236 = One Button Dialog(message=w517) -> ()  [unwired: 1 in, 1 out]
                      }
                      frame True {
                      }
                    }
                  }
                  frame #1 {
                    n237 = Greater?(x=w520, y=12.0) -> (0:w522:bool)
                    n238 = case shown="True" w522 {
                      tunnel: w524 -> [_ _]
                      tunnel: w521 -> [_ w528]
                      tunnel: w520 -> [_ w527]
                      frame False {
                      }
                      frame True {
                        n239 = Format Into String(format string="The %s is currently at %.1f C. We recommend that you contacted estates regarding this.", w528, w527) -> (resulting string=w525:string)  [unwired: 2 in, 1 out]
                        n240 = One Button Dialog(message=w525) -> ()  [unwired: 1 in, 1 out]
                      }
                    }
                  }
                }
              }
            }
            n241 = global write "Trav_pos_global.vi" "Multi Run has Inlet Heaters Enabled?"(w507) -> ()
          }
        }
      }
      frame "First Save Setup file" {
        w530 = -1 ("Currently on Row")
        n242 = global write "Trav_pos_global.vi" "Work in Tunnel Coordinates?"("Work in Tunnel Coordinates?") -> ()
        n243 = case shown="\"Run Multi Run Prog\"" w539 {
          tunnel: [w546 w548 w550 Multi_Run_Case."End" ("Multi Run Case") Multi_Run_Case."End" ("Multi Run Case")] -> w533
          tunnel: w538 -> [w546 w548 w550 _ _]
          tunnel: [w547 w549 w551 w552 w554] -> w532
          frame "Run Multi Run Prog" {
            w547 = FALSE  # Live Traverse Preview?
          }
          frame "Check Multi Run Prog With Live Moves" {
            w549 = TRUE  # Live Traverse Preview?
          }
          frame "Check Multi Run Prog" {
            w551 = FALSE  # Live Traverse Preview?
          }
          frame "Load Command File" {
            w552 = FALSE  # Live Traverse Preview?
          }
          frame "Save Command File" {
            w554 = FALSE  # Live Traverse Preview?
          }
        }
        n244 = local read "Command filename"() -> (w540:path)
        n245 = local read "Fast Plotting?"() -> (w529:bool)
        n246 = call "Save_Trav_setup.vi"("Work in Tunnel Coordinates?"="Work in Tunnel Coordinates?", "Trav Table"=w541, "Fast Plotting?"=w529, "Setup filename"=w540) -> ("Trav Table Out"=w542:T6[])  [unwired: 1 in]
        n247 = local read "Status"() -> (w535:T2)
        n248 = global write "Meas_global.vi" "Extra Comments"("") -> ()
        n249 = local write "Last Row Run"(w530) -> ()
        n250 = local write "Current Row"(w530) -> ()
        n251 = case shown="\"Continue\"" w535 {
          tunnel: [w544 Multi_Run_Case."End" ("Multi Run Case")] -> w534
          tunnel: w533 -> [w544 _]
          frame "Continue" {
          }
          frame "Jump to Next Point", Default {
          }
        }
        n252 = global write "Trav_pos_global.vi" "Live Traverse Preview?"(w532) -> ()
      }
      frame "Setup Route checking" {
        w560 = string[] []
        n253 = global read "Trav_pos_global.vi" "Work in Tunnel Coordinates?"() -> (w561:T1)
        n254 = for {
          tunnel: w564 -> [w608] mode=indexing
          shift-right: [w599] -> w562
          shift-left: string[] [] -> [w600]
          n255 = Unbundle By Name(w608) -> ("Extra Commands"=w601:string, "Start X"=w605:sgl, "Start Y"=w604:sgl, "Start Z"=w603:sgl)
          n256 = Build Array(w605, w604, w603) -> (w606:sgl[])
          n257 = Not A Number/Path/Refnum?(number/path/refnum=w606) -> (NaN/Path/Refnum?=w607:bool[])
          n258 = Not(x=w607) -> (.not. x?=w598:bool[])
          n259 = Or Array Elements(Boolean array=w598) -> (logical OR=w602:bool)
          n260 = case shown="True" w602 {
            tunnel: w601 -> [_ w613]
            tunnel: w600 -> [w609 w612]
            tunnel: [w609 w611] -> w599
            frame False {
            }
            frame True {
              n261 = call "Which_Trav_Setup.vi"("Extra Command String"=w613) -> ("Traverse Setups"=w610:string[])  [unwired: 2 out]
              n262 = Build Array (concatenate)(w612, w610) -> (w611:string[])
            }
          }
        }
        n263 = call "Analyse_string_array.vi"("String array"=w562) -> ("Unique strings"=w557:string[])  [unwired: 2 out]
        n264 = for {
          tunnel: w557 -> [w573] mode=indexing
          tunnel: w561 -> [w572]
          shift-right: [w571] -> w558
          shift-left: w560 -> [w570]
          shift-right: [w568] -> w559
          shift-left: w560 -> [w569]
          n265 = stacked-sequence {
            tunnel: w573 -> [w581 w586]
            tunnel: w572 -> [w578 _]
            tunnel: [_ w585] -> w571
            tunnel: w570 -> [_ w584]
            tunnel: w569 -> [_ w583]
            tunnel: [_ w582] -> w568
            frame #0 {
              w574 = TRUE  # Route Checking?
              w576 = TRUE  # Last Part of Move?
              n266 = call "3D_Traverse_move.vi"("Mode"=Trav_mode."Read traverse position", "Extra command String"="", "Work in Tunnel Coordinates"=w578, "Home"=Home."Don't Home", "Simulate/Run"=User_Specific_mode."Run VI", "Route Checking?"=w574, "Traverse name"=w581, "Last Part of Move?"=w576) -> ()  [unwired: 8 in, 4 out]
            }
            frame #1 {
              n267 = global read "DriveConfigGlobal.vi" "Channel Properties"() -> (w587:T23[])
              n268 = for {
                tunnel: w587 -> [w597] mode=indexing
                tunnel: w586 -> [w594]
                shift-right: [w592] -> w585
                shift-left: w584 -> [w593]
                shift-right: [w588] -> w582
                shift-left: w583 -> [w589]
                i -> [w596]
                n269 = Format Into String(format string="%d", initial string=w594, w596) -> (resulting string=w590:string)  [unwired: 1 in, 1 out]
                n270 = Unbundle By Name(w597) -> ("Metadata Ch Name"=w591:string)
                n271 = Build Array (concatenate)(w593, w591) -> (w592:string[])
                n272 = Build Array (concatenate)(w589, w590) -> (w588:string[])
              }
            }
          }
        }
        n273 = global write "Trav_pos_global.vi" "ADAM Positions Ch names"(w558) -> ()
        n274 = global write "Trav_pos_global.vi" "Route checking Chs"(w559) -> ()
        n275 = global write "Route_mapping_global.vi" "Display Mode"("Display Mode") -> ()
        n276 = global write "Trav_pos_global.vi" "Traverses to Move"(w557) -> ()
      }
      frame "Initialise Measurement Prog" {
        n277 = for {
          tunnel: w627 -> [w642] mode=indexing
          tunnel: [w640] -> w621 mode=concatenating
          tunnel: [w637] -> w617 mode=indexing
          n278 = Unbundle By Name(w642) -> ("Meas Setup File"=w641:string, "Row Type Selector"=w639:T8)
          n279 = call "Get_array_values_fr_String.vi"("String Value"=w641) -> ("String array"=w640:string[])  [unwired: 1 out]
          n280 = Equal?(x=w639, y=Multi_run_mode."Meas Fast FID Bkgnd" ("Row Type Selector")) -> (x = y?=w637:bool)
        }
        n281 = call "LDA_Mirror_Setup.vi"("Simulate/Run"=User_Specific_mode."Run VI") -> ()  [unwired: 3 in, 1 out]
        n282 = call "MultiRun Status.vi"() -> ()  [unwired: 1 in, 1 out]
        n283 = Or Array Elements(Boolean array=w617) -> (logical OR=w614:bool)
        n284 = call "Analyse_string_array.vi"("String array"=w621) -> ("Unique strings"=w620:string[])  [unwired: 1 in, 1 out]
        n285 = for {
          tunnel: w620 -> [w632] mode=indexing
          tunnel: [w632] -> w618 mode=indexing if=w631
          n286 = String Subset(string=w632, offset (0)=2, length (rest)=4 ("length (rest)")) -> (substring=w634:string)
          n287 = Not Equal?(x=w634, y="----" ("f")) -> (x != y?=w631:bool)
        }
        n288 = global write "Trav_pos_global.vi" "Measurement setup files"(w618) -> ()
        n289 = call "Perform_Meas_Setup.vi"("Simulate/Run"=User_Specific_mode."Check VI only", "String array"=w618) -> ("Continue?"=w622:bool, "FFID Bkgnd needed?"=w615:bool)
        n290 = Compound Arithmetic op=AND(w615, invert w614) -> (w616:bool)
        n291 = case shown="True" w616 {
          frame False {
          }
          frame True {
            n292 = One Button Dialog(message="This run automatically calibrates the Fast FID but does not have a Meas Fast FID Bkgnd row" ("format string")) -> ()  [unwired: 2 out]
          }
        }
        n293 = Select(t=w625, s=w622, f=Multi_Run_Case."End" ("Multi Run Case")) -> (s? t:f=w624:T3)
      }
      frame "Input Current Position" {
        n294 = call "Read_Write_Local_table_Quick.vi"("Mode"=Quick_local_ADAM_Table."Load Global From ADAM Table", "Ch names In"=string[] []) -> ()  [unwired: 1 in, 3 out]
      }
      frame "Experimental setup control" {
        # "#Check- Should this be AND?"
        n295 = global read "Trav_pos_global.vi" "Source Control?"() -> (w653:bool)
        n296 = Or(x=w653, y=w649) -> (x .or. y?=w654:bool)
        n297 = case shown="True" w654 {
          tunnel: w653 -> [_ w657]
          frame False {
          }
          frame True {
            n298 = call "Exp_Setup_Control.vi"("Source Control?"=w657) -> ()  [unwired: 3 out]
          }
        }
        n299 = global write "Trav_pos_global.vi" "FFID Background"(T6 {"Start X"=0.0, "Start Y"=0.0, "Start Z"=0.0, "End X"=0.0, "End Y"=0.0, "End Z"=0.0, "nPoints"=0, "Spacing"=enum."Linear", "Filename"=path "", "Tunnel Speed"=0.0, "Averaging time (mins)"=0.0, "Extra Commands"="", "Carrier_1 Q (l/min)"=0.0, "Carrier_2 Q (l/min)"=0.0, "Trace Gas Concentration (%)"=0.0, "Specific Arguments"="", "Comments"="", "Row No"=0, "Row Type Selector"=enum."Move Traverse Only", "EstCompl"="", "Row Duration (mins)"=0.0, "nValidPoints"=0, "Meas Setup File"=""} ("FFID Background")) -> ()
      }
      frame "Check source flowrates" {
        # "#Check- shouldn't we check source flowrates in \"Check\" mode too...?"
        n300 = case shown="\"Run VI\"" w659 {
          tunnel: w660 -> [_ w668]
          frame "Check VI only", Default {
            n301 = Get Date/Time In Seconds() -> (seconds since 1Jan1904=w666:timestamp)
            n302 = global write "Trav_pos_global.vi" "Simulation Time"(w666) -> ()
          }
          frame "Run VI" {
            n303 = global read "Trav_pos_global.vi" "Default Gas Line Name"() -> (w667:T25)
            n304 = for {
              tunnel: w668 -> [w671] mode=indexing
              tunnel: w667 -> [w670]
              n305 = call "Set_Source.vi"("Source Establishment Time (s)"=0.0, "Source Status"=Client_Source_Status."Using", "Gas Line Name"=w670, "Traverse line"=w671, "Simulate/Run"=User_Specific_mode."Check VI only") -> ()  [unwired: 6 out]
            }
          }
        }
        n306 = Increment(x=w664) -> (x+1=w661:T3)
        n307 = Select(t=w664, s=w658, f=w661) -> (s? t:f=w662:T3)
      }
      frame "Setup for running mode" {
        n308 = stacked-sequence {
          tunnel: w677 -> [w683 w692 _ _ w725 _ _ _]
          tunnel: w676 -> [_ _ _ w716 _ _ _ _]
          tunnel: [_ _ _ _ w723 _ _ _] -> w675
          frame #0 {
            n309 = for {
              tunnel: w683 -> [w689] mode=indexing
              tunnel: [w686] -> w682 mode=indexing
              n310 = Unbundle By Name(w689) -> ("Filename"=w688:path)
              n311 = Not Equal?(x=path "  ---------" ("Filename"), y=w688) -> (x != y?=w686:bool)
            }
            n312 = Or Array Elements(Boolean array=w682) -> (logical OR=w681:bool)
            n313 = case shown="True" w681 {
              tunnel: [FALSE ("Send Emails? 2") w685] -> w680
              frame False {
              }
              frame True {
                n314 = call "MultiRun Description.vi"() -> ("Send Emails? Out"=w685:bool)  [unwired: 11 in]
              }
            }
            n315 = global write "Preference_global.vi" "Send Emails?"(w680) -> ()
          }
          frame #1 {
            n316 = for {
              tunnel: w692 -> [w696] mode=indexing
              tunnel: [w693] -> w691 mode=indexing
              n317 = Unbundle By Name(w696) -> ("Row Type Selector"=w695:T8)
              n318 = Equal?(x=Multi_run_mode."Synchronize With:" ("Row Type Selector"), y=w695) -> (x = y?=w693:bool)
            }
            n319 = call "Setup_Environment.vi"() -> ()  [unwired: 1 in, 1 out]
            n320 = Or Array Elements(Boolean array=w691) -> (logical OR=w690:bool)
            n321 = case shown="True" w690 {
              frame False {
              }
              frame True {
                n322 = call "Declare_Sync_Client.vi"() -> ()  [unwired: 6 out]
              }
            }
          }
          frame #2 {
            n323 = Open VI Reference(vi path="Display_Trav_Views.vi" ("VI path")) -> (vi reference=w702:refnum<vi>, error out=w701:errorcluster)  [unwired: 1 in, 4 out]
            n324 = property class="VI"(reference=w702, error in=w701, "Front Panel Window:Open"=FALSE) -> (reference out=w699:refnum<vi>, error out=w698:errorcluster)
            n325 = global write "Meas_global.vi" "Post Process"(Post_Process."Take New Data" ("Post Process")) -> ()
            n326 = Close Reference(reference=w699, error in (no error)=w698) -> ()  [unwired: 1 out]
          }
          frame #3 {
            w708 = 36000.0  # 10 Hours
            w711 = TRUE  # Start of Multi Run Prog
            n327 = Get Date/Time In Seconds() -> (seconds since 1Jan1904=w710:timestamp)
            n328 = feedback #1() -> (w704:dbl)  [unwired: 1 in]
            n329 = To Double Precision Float(number=w710) -> (double precision float=w705:dbl)
            n330 = global write "Meas_global.vi" "Start Time of experiment"(w705) -> ()
            n331 = Subtract(x=w705, y=w704) -> (x-y=w709:dbl)
            n332 = Greater?(x=w709, y=w708) -> (0:w707:bool)
            n333 = local read "Command filename"() -> (w715:path)
            n334 = case shown="True" w707 {
              tunnel: [w717 w719] -> w706
              tunnel: w705 -> [_ w719]
              tunnel: w704 -> [w717 _]
              frame False {
              }
              frame True {
                n335 = global write "Preference_global.vi" "Unblock Email"(TRUE) -> ()
              }
            }
            n336 = feedback-in #1(w706) -> ()
            n337 = Path To String(path=w715) -> (string=w713:string)
            n338 = Concatenate Strings("Commencing a new multi run Prog having the setup filename of :" ("Message"), w713) -> (w712:string)
            n339 = call "Log_Current_row_to_Execute.vi"("Simulate/Run"=w716, "Message"=w712, "Start of Multi Run Prog"=w711) -> ()  [unwired: 2 in, 5 out]
          }
          frame #4 {
            n340 = call "Calc_Remaining_Time.vi"("Table In"=w725, "Currently on Row"=-1) -> ("Table Out"=w723:T6[], "Estimated Completion time"=w722:string, "noWaitCompletion"=w721:timestamp, "remainingTime"=w720:string)
            n341 = local write "remainingTime"(w720) -> ()
            n342 = global write "Trav_pos_global.vi" "Estimated Completion time"(w722) -> ()
            n343 = local write "PredictedEnd"(w721) -> ()
            n344 = local write "Estimated Completion"(w722) -> ()
          }
          frame #5 {
            n345 = global read "Preference_global.vi" "Rig Setup"() -> (w726:string)
            n346 = case shown="\"EnFlo_Tunnel\"" w726 {
              frame Default {
              }
              frame "EnFlo_Tunnel" {
                w731 = "EnFlo_Tunnel:Inlet:Conditioning"
                n347 = call "Get_Current_Scan_client.vi"("singleChannel"=w731) -> ("Numerical Values"=w733:dbl[])  [unwired: 1 in, 3 out]
                n348 = Index Array(array=w733) -> (element=w734:dbl)  [unwired: 1 in]
                n349 = Greater Than 0?(x=w734) -> (x > 0?=w729:bool)
                n350 = call "Get_Current_Scan_client.vi"("singleChannel"="GMU:Source:Live") -> ("Numerical Values"=w738:dbl[])  [unwired: 1 in, 3 out]
                n351 = case shown="True" w729 {
                  tunnel: "Is not on. Do you want to turn it on?" ("string") -> [w744 _]
                  tunnel: w731 -> [w741 _]
                  tunnel: [w740 FALSE ("T button?")] -> w730
                  frame False {
                    n352 = Concatenate Strings(w741, w744) -> (w745:string)
                    n353 = Two Button Dialog(message=w745, 1:"No" ("F button name (\"Cancel\")"), 2:"Yes" ("T button name (\"OK\")")) -> (T button?=w740:bool)
                  }
                  frame True {
                  }
                }
                n354 = Index Array(array=w738) -> (element=w737:dbl)  [unwired: 1 in]
                n355 = Greater?(x=w737, y=0.5) -> (0:w735:bool)
                n356 = global write "Gas_management_global.vi" "Source Live"(w735) -> ()
                n357 = case shown="False" w730 {
                  tunnel: w731 -> [_ w749]
                  frame False {
                  }
                  frame True {
                    n358 = Build Array(w749) -> (w750:string[])
                    n359 = Build Array(1.0) -> (w747:dbl[])
                    n360 = call "ASYNC_Adam_client.vi"("Values"=w747, "Channel Names"=w750) -> ()  [unwired: 1 in, 2 out]
                  }
                }
              }
              frame "Aero_Tunnel" {
                n361 = call "Get_Current_Scan_client.vi"("singleChannel"="GMU2:Source:Live") -> ("Numerical Values"=w754:dbl[])  [unwired: 1 in, 3 out]
                n362 = Index Array(array=w754) -> (element=w753:dbl)  [unwired: 1 in]
                n363 = Greater?(x=w753, y=0.5) -> (0:w751:bool)
                n364 = global write "Gas_management_global.vi" "Source Live"(w751) -> ()
              }
            }
            n365 = call "Program_Active_Client.vi"("Mode"=enum16{"Program Active", "Traverse Level State"}."Traverse Level State", "Traverse level State"=Traverse_Level_State."Running") -> ()  [unwired: 1 in, 3 out]
          }
          frame #6 {
            n366 = case shown="True" "Fast Plotting?" {
              frame False {
              }
              frame True {
                n367 = Two Button Dialog(message="Fast Plotting? is set to True. This will disable all the backlash moves\nand keep the traverse motors alive during the whole run.", 1:"Turn off Fast Plotting" ("F button name (\"Cancel\")"), 2:"Continue" ("T button name (\"OK\")")) -> (T button?=w757:bool)
                n368 = case shown="False" w757 {
                  frame False {
                    n369 = local write "Fast Plotting?"(FALSE ("Fast Plotting?")) -> ()
                  }
                  frame True {
                  }
                }
              }
            }
          }
          frame #7 {
            n370 = local read "Fast Plotting?"() -> (w764:bool)
            n371 = global write "Meas_global.vi" "Error handler Log"("") -> ()
            n372 = global write "Trav_pos_global.vi" "MultiRun Has Jumped?"(FALSE ("MultiRun Has Jumped?")) -> ()
            n373 = global write "Trav_pos_global.vi" "Fast Plotting?"(w764) -> ()
          }
        }
      }
      frame "Skip Blank Rows" {
        n374 = stacked-sequence {
          tunnel: w769 -> [w772 w795]
          tunnel: w766 -> [w770 w792]
          frame #0 {
            n375 = Decrement(x=w772) -> (x-1=w771:i32)
            n376 = while {
              tunnel: w770 -> [w782]
              tunnel: w771 -> [w776]
              stop <- w773 continue-if-true
              n377 = local read "Current Row"() -> (w778:i32)
              n378 = Increment(x=w778) -> (x+1=w777:i32)
              n379 = Index Array(array=w782, index=w777) -> (element=w781:T6)
              n380 = Less?(x=w777, y=w776) -> (x < y?=w775:bool)
              n381 = Unbundle By Name(w781) -> ("Row Type Selector"=w780:T8)
              n382 = Equal?(x=Multi_run_mode."Blank Row" ("Row Type Selector"), y=w780) -> (x = y?=w774:bool)
              n383 = And(x=w774, y=w775) -> (x .and. y?=w773:bool)
              n384 = case shown="True" w774 {
                tunnel: w777 -> [_ w783]
                frame False {
                }
                frame True {
                  n385 = local write "Current Row"(w783) -> ()
                }
              }
            }
          }
          frame #1 {
            n386 = local read "Progress"() -> (w785:i32)
            n387 = local read "Current Row"() -> (w787:i32)
            n388 = Not Equal To 0?(x=w787) -> (x != 0?=w788:bool)
            n389 = Increment(x=w787) -> (x+1=w784:i32)
            n390 = Select(t=w784, s=w788, f=w785) -> (s? t:f=→"Progress":i32)
            n391 = Increment(x=w787) -> (x+1=w793:i32)
            n392 = Index Array(array=w792, index=w793) -> (element=w794:T6)
            n393 = Unbundle By Name(w794) -> ("Row Type Selector"=w791:T8)
            n394 = Equal?(x=Multi_run_mode."Turn Off Row Repeating" ("Row Type Selector"), y=w791) -> (x = y?=w789:bool)
            n395 = while {
              shift-right: [w804] -> _
              shift-left: _ -> [w803]
              tunnel: w795 -> [w800]
              tunnel: w787 -> [w804]
              tunnel: w789 -> [w797]
              stop <- TRUE stop-if-true
              n396 = Decrement(x=w800) -> (x-1=w805:i32)
              n397 = Equal?(x=w804, y=w805) -> (x = y?=w798:bool)
              n398 = Not Equal?(x=w804, y=w803) -> (x != y?=w802:bool)
              n399 = Or(x=w797, y=w798) -> (x .or. y?=w796:bool)
              n400 = And(x=w802, y=w796) -> (x .and. y?=w801:bool)
              n401 = case shown="True" w801 {
                tunnel: w800 -> [_ w806]
                frame False {
                }
                frame True {
                  n402 = Initialize Array(timestamp(0 s since 1904-01-01) ("seconds since 1Jan1904"), w806) -> (w808:timestamp[])
                  n403 = global write "Trav_pos_global.vi" "Row completion times"(w808) -> ()
                }
              }
            }
          }
        }
      }
      frame "Which row to execute next" {
        # "last"
        # "Repeat\nRow"
        n404 = local read "Current Row"() -> (w809:i32)
        n405 = stacked-sequence {
          seq-local: [_ w838 _ _] -> [_ _ w875 _]
          seq-local: [_ w837 _ _] -> [_ _ w876 _]
          seq-local: [w818 _ _ _] -> [_ w836 _ _]
          seq-local: [_ w833 _ _] -> [_ _ w869 _]
          tunnel: [w821 _ _ _] -> w815
          tunnel: w814 -> [w821 w840 w883 _]
          tunnel: w813 -> [_ _ w881 _]
          tunnel: w812 -> [_ w835 w882 w912]
          tunnel: [_ _ w878 _] -> w811
          tunnel: w810 -> [_ _ w877 _]
          tunnel: w809 -> [w822 w832 w868 _]
          frame #0 {
            n406 = Increment(x=w822) -> (x+1=w820:i32)
            n407 = for {
              N: w820 -> [_]
              tunnel: w821 -> [w831] mode=indexing
              shift-right: [w828] -> w818
              shift-left: -1 -> [w825]
              i -> [w826]
              n408 = Unbundle By Name(w831) -> ("Row Type Selector"=w830:T8)
              n409 = Equal?(x=Multi_run_mode."Turn Off Row Repeating" ("Row Type Selector"), y=w830) -> (x = y?=w827:bool)
              n410 = Select(t=w826, s=w827, f=w825) -> (s? t:f=w828:i32)
            }
            n411 = global write "Trav_pos_global.vi" "Currently on point"(0 ("Currently on point")) -> ()
            n412 = global write "Trav_pos_global.vi" "Paused During Row?"(FALSE ("Paused During Row?")) -> ()
          }
          frame #1 {
            n413 = global read "Trav_pos_global.vi" "Row completion times"() -> (w839:timestamp[])
            n414 = global read "Extra_Commands_Global.vi" "Minutes Before Repeating Row"() -> (w834:string)
            n415 = case shown="\"Run VI\"" w835 {
              tunnel: [w841 w842] -> w833
              frame "Check VI only" {
                n416 = global read "Trav_pos_global.vi" "Simulation Time"() -> (w841:timestamp)
              }
              frame "Run VI" {
                n417 = Get Date/Time In Seconds() -> (seconds since 1Jan1904=w842:timestamp)
                n418 = global write "Trav_pos_global.vi" "Simulation Time"(w842) -> ()
              }
            }
            n419 = while {
              tunnel: w840 -> [w853] mode=indexing
              tunnel: w839 -> [w856]
              tunnel: w833 -> [w855]
              tunnel: [w847] -> w838
              tunnel: [w845] -> w837
              tunnel: w836 -> [w844]
              tunnel: w832 -> [w848]
              tunnel: w834 -> [w846]
              i -> [w845]
              stop <- w852 continue-if-true
              n420 = Unbundle By Name(w853) -> ("Extra Commands"=w857:string)
              n421 = call "Extra_Commands.vi"("String to Search"=w857, "Command"=w846) -> ("Numeric Value"=w854:dbl, "Command Found"=w850:bool)  [unwired: 1 in, 3 out]
              n422 = Greater?(x=w845, y=w844) -> (0:w843:bool)
              n423 = And(x=w843, y=w850) -> (x .and. y?=w849:bool)
              n424 = case shown="True" w849 {
                tunnel: w856 -> [_ w863]
                tunnel: w855 -> [_ w864]
                tunnel: w845 -> [_ w862]
                tunnel: w854 -> [_ w860]
                tunnel: [FALSE w859] -> w847
                frame False {
                }
                frame True {
                  n425 = Index Array(array=w863, index=w862) -> (element=w865:timestamp)
                  n426 = Subtract(x=w864, y=w865) -> (x-y=w866:dbl)
                  n427 = Divide(x=w866, y=60.0) -> (x/y=w861:dbl)
                  n428 = Greater?(x=w861, y=w860) -> (0:w859:bool)
                }
              }
              n429 = Less?(x=w845, y=w848) -> (x < y?=w851:bool)
              n430 = Compound Arithmetic op=AND(invert w847, w851) -> (w852:bool)
            }
          }
          frame #2 {
            n431 = Not Equal?(x=w868, y=w876) -> (x != y?=w874:bool)
            n432 = And(x=w875, y=w874) -> (x .and. y?=w873:bool)
            n433 = case shown="True" w873 {
              tunnel: w876 -> [_ w909]
              tunnel: w868 -> [w905 w910]
              tunnel: [w904 w908] -> w879
              tunnel: [w904 w909] -> w870
              tunnel: w881 -> [w907 _]
              tunnel: [w903 TRUE] -> w880
              frame False {
                n434 = Increment(x=w905) -> (x+1=w906:i32)
                n435 = Greater?(x=w907, y=w906) -> (0:w903:bool)
                n436 = Select(t=w906, s=w903, f=w905) -> (s? t:f=w904:i32)
              }
              frame True {
                n437 = Max & Min(x=w910, y=w909) -> (max(x,y)=w908:i32)  [unwired: 1 out]
              }
            }
            n438 = global read "Trav_pos_global.vi" "Row completion times"() -> (w872:timestamp[])
            n439 = case shown="True" w880 {
              tunnel: w870 -> [_ w891]
              tunnel: w883 -> [_ w897]
              tunnel: w882 -> [w885 w889]
              tunnel: w879 -> [_ w895]
              tunnel: [w884 w894] -> w878
              tunnel: w877 -> [_ w894]
              frame False {
                n440 = case shown="\"Run VI\"" w885 {
                  tunnel: [Multi_Run_Case."Show jumped positions" ("Multi Run Case") Multi_Run_Case."Shut down source etc" ("Multi Run Case")] -> w884
                  frame "Check VI only" {
                  }
                  frame "Run VI" {
                  }
                }
              }
              frame True {
                n441 = Index Array(array=w897, index=w891) -> (element=w893:T6)
                n442 = Bundle By Name(cluster=w893, "Row No"=w891) -> (w892:T6)
                n443 = Build Array(w895) -> (w896:i32[])
                n444 = global write "Trav_pos_global.vi" "Meas Setup Number"(0 ("Meas Setup Number")) -> ()
                n445 = property on="Table" class="Arr (strict)"("Index Values"=w896) -> ()  [unwired: 2 in, 2 out]
                n446 = case shown="\"Check VI only\"" w889 {
                  selector: w889 -> [_ w899]
                  tunnel: w892 -> [w898 w901]
                  tunnel: [w898 w900] -> w888
                  frame "Check VI only" {
                  }
                  frame "Run VI" {
                    n447 = call "Log_Current_row_to_Execute.vi"("Simulate/Run"=w899, "Start of Multi Run Prog"=FALSE, "Traverse line in"=w901) -> ("Traverse line Out"=w900:T6)  [unwired: 2 in, 4 out]
                  }
                }
                n448 = global write "Trav_pos_global.vi" "Current Row"(w888) -> ()
                "Current Row" <- w895
              }
            }
            n449 = Replace Array Subset(array=w872, new element=w869, index=w870) -> (w871:timestamp[])
            n450 = global write "Trav_pos_global.vi" "Row completion times"(w871) -> ()
          }
          frame #3 {
            n451 = case shown="\"Check VI only\"" w912 {
              frame "Check VI only" {
              }
              frame "Run VI" {
                n452 = disable-structure shown="Disabled" {
                  frame Disabled {
                    w922 = 28800.0  # 8 Hours in seconds
                    # "Restarts the camera server ever 8 hours of running."
                    n453 = global read "Meas_global.vi" "Start Time of experiment"() -> (w925:dbl)
                    n454 = Get Date/Time In Seconds() -> (seconds since 1Jan1904=w926:timestamp)
                    n455 = To Double Precision Float(number=w926) -> (double precision float=w924:dbl)
                    n456 = Subtract(x=w924, y=w925) -> (x-y=w923:dbl)
                    n457 = global read "Preference_global.vi" "Rig Setup"() -> (w916:string)
                    n458 = Quotient & Remainder(x=w923, y=w922) -> (floor(x/y)=w920:dbl)  [unwired: 1 out]
                    n459 = Greater Than 0?(x=w920) -> (x > 0?=w918:bool)
                    n460 = Equal?(x=w916, y="EnFlo_Tunnel") -> (x = y?=w915:bool)
                    n461 = global read "Preference_global.vi" "Log Cameras if available"() -> (w914:bool)
                    n462 = feedback #2() -> (w921:dbl)  [unwired: 1 in]
                    n463 = feedback-in #2(w920) -> ()
                    n464 = Not Equal?(x=w920, y=w921) -> (x != y?=w919:bool)
                    n465 = Compound Arithmetic op=AND(w919, w918, w915, w914) -> (w913:bool)
                    n466 = case shown="True" w913 {
                      frame False {
                      }
                      frame True {
                        n467 = flat-sequence {
                          frame #0 {
                            n468 = call "Remote Restart Camera server.vi"() -> ()  [unwired: 1 out]
                          }
                          frame #1 {
                            n469 = call "Wait_Seconds_with_display.vi"("Message"="Restarting Camera Server", "Seconds to wait"=120.0) -> ()  [unwired: 1 in, 1 out]
                          }
                        }
                      }
                    }
                  }
                  frame Enabled {
                  }
                }
              }
            }
          }
        }
      }
      frame "Evaluate IF Statement" {
        n470 = global read "Trav_pos_global.vi" "Current Row"() -> (w933:T6)
        n471 = Unbundle By Name(w933) -> ("Extra Commands"=w934:string)
        n472 = global read "Extra_Commands_Global.vi" "If Command"() -> (w937:string)
        n473 = call "Extra_Commands.vi"("String to Search"=w934, "Command"=w937) -> ("String Value"=w936:string, "Command Found"=w930:bool)  [unwired: 1 in, 3 out]
        n474 = And(x=w929, y=w930) -> (x .and. y?=w931:bool)
        n475 = case shown="True" w931 {
          tunnel: w936 -> [_ w947]
          tunnel: [w943 w946] -> w932
          frame False {
            w943 = TRUE  # Execute Row?
          }
          frame True {
            n476 = call "Get_array_values_fr_String.vi"("String Value"=w947) -> ("Numeric Array"=w945:dbl[], "String array"=w944:string[])
            n477 = Index Array(array=w944, index=0 ("Index")) -> (element=w948:string)
            n478 = case shown="\"Time Between\"" w948 {
              tunnel: w947 -> [w953 _ _ _]
              tunnel: [w952 w954 w965 TRUE ("Execute Row?")] -> w946
              tunnel: w945 -> [_ w960 w977 _]
              tunnel: w944 -> [_ _ w971 _]
              frame "Time Between" {
                n479 = Get Date/Time In Seconds() -> (seconds since 1Jan1904=w950:timestamp)
                n480 = To Double Precision Float(number=w950) -> (double precision float=w951:dbl)
                n481 = call "If_Time_arguments.vi"("seconds since 1Jan1904"=w951, "String Value"=w953) -> ("Execute Row?"=w952:bool)  [unwired: 2 out]
              }
              frame "Global Value Between" {
                n482 = global read "Extra_Commands_Global.vi" "If command global value"() -> (w955:dbl)
                n483 = Index Array(array=w960, index=1 ("Index")) -> (element=w958:dbl)
                n484 = Index Array(array=w960, index=2 ("Index")) -> (element=w959:dbl)
                n485 = Max & Min(x=w958, y=w959) -> (max(x,y)=w957:dbl, min(x,y)=w956:dbl)
                n486 = In Range and Coerce(upper limit=w957, x=w955, lower limit=w956) -> (In Range?=w954:bool)  [unwired: 1 out]
              }
              frame "ADAM Channel Between" {
                n487 = Index Array(array=w971, index=1 ("Index")) -> (element=w963:string)
                n488 = Index Array(array=w977, index=2 ("Index")) -> (element=w975:dbl)
                n489 = Index Array(array=w977, index=3 ("Index")) -> (element=w976:dbl)
                n490 = Max & Min(x=w975, y=w976) -> (max(x,y)=w974:dbl, min(x,y)=w973:dbl)
                n491 = call "Get_Current_Scan_client.vi"("singleChannel"=w963) -> ("Numerical Values"=w969:dbl[])  [unwired: 1 in, 3 out]
                n492 = Index Array(array=w969, index=0 ("Index")) -> (element=w968:dbl)
                n493 = In Range and Coerce(upper limit=w974, x=w968, lower limit=w973) -> (In Range?=w966:bool)  [unwired: 1 out]
                n494 = Not A Number/Path/Refnum?(number/path/refnum=w968) -> (NaN/Path/Refnum?=w967:bool)
                n495 = Select(t=TRUE, s=w967, f=w966) -> (s? t:f=w965:bool)
              }
              frame "No Match", Default {
              }
            }
          }
        }
        n496 = Select(t=w940, s=w932, f=Multi_Run_Case."Calculate Row TIme" ("Multi Run Case")) -> (s? t:f=w939:T3)
      }
      frame "Perform Measurement Setup" {
        n497 = global read "Trav_pos_global.vi" "Current Row"() -> (w983:T6)
        n498 = case shown="\"Run VI\"" w982 {
          selector: w982 -> [_ w987]
          tunnel: w983 -> [_ w988]
          frame "Check VI only" {
          }
          frame "Run VI" {
            n499 = stacked-sequence {
              tunnel: w988 -> [w991 _]
              tunnel: w987 -> [w989 _]
              frame #0 {
                n500 = Unbundle By Name(w991) -> ("Extra Commands"=w990:string)
                n501 = call "Pause_for_server_ch_val.vi"("Extra command string"=w990, "Simulate/Run"=w989) -> ()  [unwired: 2 out]
              }
              frame #1 {
                n502 = Get Date/Time In Seconds() -> (seconds since 1Jan1904=w992:timestamp)
                n503 = To Double Precision Float(number=w992) -> (double precision float=w993:dbl)
                n504 = global write "Trav_pos_global.vi" "Start of Row time (Sec)"(w993) -> ()
              }
            }
          }
        }
      }
      frame "Set Measurement Conditions" {
        w1000 = TRUE  # Row Completed
        w999 = FALSE  # Row Completed
        n505 = global read "Trav_pos_global.vi" "Current Row"() -> (w997:T6)
        n506 = Unbundle By Name(w997) -> ("Row Type Selector"=w1002:T8)
        n507 = global read "Preference_global.vi" "Default Source Establishment Time (s)"() -> (w994:dbl)
        n508 = case shown="\"Run VI Named:\"" w1002 {
          tunnel: [TRUE FALSE TRUE TRUE TRUE TRUE FALSE FALSE TRUE FALSE w1048 FALSE FALSE FALSE] -> w1007
          tunnel: w997 -> [w1015 w1018 w1021 w1024 w1027 w1030 w1033 w1036 w1039 w1041 w1047 w1069 w1072 w1077]
          tunnel: [w1015 w1018 w1021 w1024 w1027 w1030 w1033 w1036 w1039 w1041 w1046 w1069 w1072 w1077] -> w1003
          tunnel: [w1014 w1017 w1020 w1023 w1026 w1029 w1032 w1035 w1038 w1042 w1045 w1068 w1074 w1076] -> w1001
          tunnel: w1000 -> [w1014 _ w1020 w1023 w1026 _ _ _ _ _ w1045 w1068 w1074 w1076]
          tunnel: w999 -> [_ w1017 _ _ _ w1029 w1032 w1035 w1038 w1042 _ _ _ _]
          tunnel: w995 -> [_ _ _ _ _ _ _ _ _ _ w1044 _ _ _]
          frame "Move Traverse Only" {
          }
          frame "Check Beam Power" {
          }
          frame "Set Tunnel Speed Only" {
          }
          frame "Set Source Only" {
          }
          frame "Set Measurement Conditions" {
          }
          frame "Single Measurement" {
          }
          frame "Vertical Profile", Default {
          }
          frame "Jump to Fall Back Row" {
          }
          frame "Scanning Valve Measurement" {
          }
          frame "Run VI Named:" {
          }
          frame "Send Message" {
            n509 = stacked-sequence {
              tunnel: [_ _ FALSE] -> w1048
              tunnel: w1047 -> [w1056 w1062 w1065]
              tunnel: [_ _ w1065] -> w1046
              tunnel: w1044 -> [w1049 _ _]
              frame #0 {
                n510 = Unbundle By Name(w1056) -> ("Specific Arguments"=w1051:string, "Comments"=w1052:string, "Filename"=w1054:path)
                n511 = Concatenate Strings(w1051, w1052) -> (w1050:string)
                n512 = Build Array(w1054) -> (w1053:path[])
                n513 = case shown="\"Check VI only\", Default" w1049 {
                  tunnel: "Message" ("Error Type") -> [_ w1059]
                  tunnel: w1050 -> [_ w1058]
                  tunnel: w1053 -> [_ w1057]
                  frame "Check VI only", Default {
                  }
                  frame "Run VI" {
                    n514 = call "Email_Text_Files.vi"("Filenames"=w1057, "message"=w1058, "subject ([No Subject])"=w1059) -> ()
                  }
                }
              }
              frame #1 {
                n515 = Unbundle By Name(w1062) -> ("Extra Commands"=w1063:string)
                n516 = global read "Extra_Commands_Global.vi" "Establish Exp Conditions (s)"() -> (w1064:string)
                n517 = call "Extra_Commands.vi"("String to Search"=w1063, "Command"=w1064) -> ("Numeric Value"=w1060:dbl)  [unwired: 1 in, 4 out]
                n518 = call "Wait_Seconds_with_display.vi"("Message"="In Send Message Row", "Seconds to wait"=w1060) -> ()  [unwired: 2 out]
              }
              frame #2 {
              }
            }
          }
          frame "Fall Back to this Row" {
          }
          frame "Turn Off Row Repeating" {
            n519 = Bundle By Name(cluster=w1072, "Row Type Selector"=Multi_run_mode."Blank Row") -> (w1071:T6)
            n520 = global write "Trav_pos_global.vi" "FFID Background"(w1071) -> ()
          }
          frame "Blank Row" {
          }
        }
        n521 = case shown="False" w1007 {
          tunnel: w1003 -> [_ w1081]
          tunnel: w995 -> [_ w1085]
          tunnel: [Multi_Run_Status."Continue" ("Status") w1082] -> w996
          tunnel: w994 -> [_ w1079]
          frame False {
          }
          frame True {
            w1084 = 1  # Currently on Point
            n522 = global read "Trav_pos_global.vi" "Default Gas Line Name"() -> (w1080:T25)
            n523 = call "Set_Measurement_Conditions.vi"("Traverse line"=w1081, "Gas Line Name"=w1080, "Currently on Point"=w1084, "Simulate/Run"=w1085, "Source Establishment Time (s)"=w1079) -> ("Status Cluster"=w1083:T26)  [unwired: 2 in]
            n524 = Unbundle By Name(w1083) -> ("Status"=w1082:T2)
            n525 = call "Program_Active.vi"() -> ()  [unwired: 1 in]
          }
        }
        n526 = case shown="\"Jump to Next Point\", Default" w996 {
          tunnel: [w1011 Multi_Run_Case."Calculate Row TIme" ("Multi Run Case")] -> w1006
          tunnel: w1005 -> [w1012 _]
          tunnel: w1001 -> [w1009 _]
          frame "Continue", "Continue with Error" {
            n527 = Select(t=Multi_Run_Case."Calculate Row TIme" ("Multi Run Case"), s=w1009, f=w1012) -> (s? t:f=w1011:T3)
          }
          frame "Jump to Next Point", Default {
          }
        }
        n528 = local write "Status"(w996) -> ()
      }
      frame "Execute Row" {
        n529 = global read "Trav_pos_global.vi" "Current Row"() -> (w1087:T6)
        n530 = stacked-sequence {
          tunnel: w1088 -> [w1092 w1103 w1106]
          tunnel: w1087 -> [w1093 w1100 w1105]
          frame #0 {
            n531 = case shown="\"Check VI only\"" w1092 {
              selector: w1092 -> [w1094 _]
              tunnel: w1093 -> [w1096 _]
              frame "Check VI only" {
                n532 = Unbundle By Name(w1096) -> ("Extra Commands"=w1097:string, "Row No"=w1099:i32, "Meas Setup File"=w1095:string)
                n533 = call "Skip_If Sd_Error_Below.vi"("String to Search"=w1097, "Simulate/Run"=w1094, "Measurement setup Applied?"=TRUE, "Row Number"=w1099, "Measurement Setup File"=w1095) -> ()  [unwired: 5 out]
              }
              frame "Run VI" {
              }
            }
          }
          frame #1 {
            n534 = call "Execute_Row.vi"("Simulate/Run"=w1103, "Traverse line"=w1100) -> ("Status"=w1102:T2, "Traverse line out"=w1101:T6)  [unwired: 2 out]
            n535 = local write "Status"(w1102) -> ()
            n536 = global write "Trav_pos_global.vi" "Current Row"(w1101) -> ()
          }
          frame #2 {
            w1109 = FALSE  # Empty list
            n537 = call "Remember_RD_Folders.vi"("Empty list"=w1109) -> ("List of Folders"=w1108:path[])  [unwired: 1 in]
            n538 = for {
              tunnel: w1105 -> [w1118]
              tunnel: w1108 -> [w1111] mode=indexing
              tunnel: "Muti_Run_Log.xls" ("name or relative path") -> [w1117]
              tunnel: w1106 -> [w1116]
              tunnel: "Extra Info" ("name or relative path") -> [w1114]
              n539 = Strip Path(path=w1111) -> (stripped path=w1110:path)  [unwired: 1 out]
              n540 = Build Path(base path=w1110, name or relative path=w1114) -> (appended path=w1115:path)
              n541 = Build Path(base path=w1115, name or relative path=w1117) -> (appended path=w1113:path)
              n542 = call "Create_directory_path.vi"("Path name"=w1113) -> ("Path name Out"=w1112:path)  [unwired: 2 in, 1 out]
              n543 = call "Log_Current_row_to_Execute.vi"("Simulate/Run"=w1116, "Start of Multi Run Prog"=FALSE, "Traverse line in"=w1118, "Multi Run Log File"=w1112) -> ()  [unwired: 1 in, 5 out]
            }
          }
        }
      }
      frame "Calculate Row TIme" {
        n544 = global read "Trav_pos_global.vi" "Paused During Row?"() -> (w1124:bool)
        n545 = local read "Status"() -> (w1126:T2)
        n546 = global read "Trav_pos_global.vi" "Current Row"() -> (w1123:T6)
        n547 = Less?(x=w1126, y=Multi_Run_Status."Jump to Next Point" ("Status")) -> (x < y?=w1125:bool)
        n548 = Compound Arithmetic op=AND(w1125, w1120, invert w1124) -> (w1122:bool)
        n549 = case shown="False" w1122 {
          tunnel: w1123 -> [w1139 w1150]
          frame False {
            n550 = global read "Trav_pos_global.vi" "Simulation Time"() -> (w1140:timestamp)
            n551 = To Double Precision Float(number=w1140) -> (double precision float=w1134:dbl)
            n552 = call "Calculate_Row_Time.vi"("Multi Run Row"=w1139, "Row Start Time (Sec Since 1904)"=w1134) -> ("Fixed Time (Sec)"=w1135:dbl, "Scalable Time (Sec)"=w1137:dbl)  [unwired: 1 out]
            n553 = call "Overhead_Factor.vi"("Mode"=Overhead."Read Current Overhead") -> ("Current Overhead Factor"=w1138:dbl)  [unwired: 3 in]
            n554 = Multiply(x=w1137, y=w1138) -> (x*y=w1136:dbl)
            n555 = Add(x=w1135, y=w1136) -> (x+y=w1132:dbl)
            n556 = Add(x=w1134, y=w1132) -> (x+y=w1131:dbl)
            n557 = global write "Trav_pos_global.vi" "Start of Row time (Sec)"(w1132) -> ()
            n558 = To Time Stamp(1:w1131) -> (0:w1133:timestamp)
            n559 = global write "Trav_pos_global.vi" "Simulation Time"(w1133) -> ()
          }
          frame True {
            n560 = global read "Trav_pos_global.vi" "Start of Row time (Sec)"() -> (w1148:dbl)
            n561 = Get Date/Time In Seconds() -> (seconds since 1Jan1904=w1143:timestamp)
            n562 = To Double Precision Float(number=w1143) -> (double precision float=w1142:dbl)
            n563 = call "Calculate_Row_Time.vi"("Multi Run Row"=w1150, "Row Start Time (Sec Since 1904)"=w1148) -> ("Fixed Time (Sec)"=w1146:dbl, "Scalable Time (Sec)"=w1144:dbl)  [unwired: 1 out]
            n564 = Subtract(x=w1142, y=w1148) -> (x-y=w1147:dbl)
            n565 = Subtract(x=w1147, y=w1146) -> (x-y=w1145:dbl)
            n566 = call "Overhead_Factor.vi"("Sum of Ideal times (Sec)"=w1144, "Sum of Actual times (Sec)"=w1145, "Mode"=Overhead."Update total times") -> ()  [unwired: 1 in, 1 out]
          }
        }
      }
      frame "Update time estimate" {
        n567 = global read "Trav_pos_global.vi" "Current Row"() -> (w1154:T6)
        n568 = local read "Current Row"() -> (w1153:i32)
        n569 = Unbundle By Name(w1154) -> ("Row No"=w1152:i32)
        n570 = Equal?(x=w1152, y=w1153) -> (x = y?=w1151:bool)
        n571 = case shown="\"Run VI\"" w1157 {
          tunnel: w1160 -> [w1165 w1190]
          tunnel: [w1169 w1186] -> w1159
          tunnel: w1156 -> [_ w1192]
          tunnel: [w1164 w1191] -> w1155
          tunnel: w1153 -> [w1167 w1185]
          tunnel: w1154 -> [w1168 w1189]
          tunnel: w1151 -> [w1166 w1188]
          frame "Check VI only" {
            n572 = global read "Trav_pos_global.vi" "Simulation Time"() -> (w1163:timestamp)
            n573 = call "timestampISO8601String.vi"("Time Stamp"=w1163) -> ("date/time"=w1164:string)  [unwired: 5 in, 5 out]
            n574 = case shown="True" w1166 {
              tunnel: w1167 -> [_ w1179]
              tunnel: [w1170 w1177] -> w1169
              tunnel: w1164 -> [_ w1176]
              tunnel: w1168 -> [_ w1175]
              tunnel: w1165 -> [w1170 w1171]
              frame False {
              }
              frame True {
                n575 = global read "Trav_pos_global.vi" "Start of Row time (Sec)"() -> (w1174:dbl)
                n576 = Divide(x=w1174, y=60.0) -> (x/y=w1172:dbl)
                n577 = Bundle By Name(cluster=w1175, "EstCompl"=w1176, "Row Duration (mins)"=w1172) -> (w1178:T6)
                n578 = Replace Array Subset(array=w1171, new element=w1178, index=w1179) -> (w1177:T6[])
              }
            }
          }
          frame "Run VI" {
            n579 = case shown="True" w1188 {
              tunnel: w1185 -> [_ w1200]
              tunnel: w1190 -> [w1196 w1199]
              tunnel: w1189 -> [_ w1198]
              tunnel: [w1196 w1197] -> w1187
              frame False {
              }
              frame True {
                n580 = Replace Array Subset(array=w1199, new element=w1198, index=w1200) -> (w1197:T6[])
              }
            }
            n581 = call "Calc_Remaining_Time.vi"("Table In"=w1187, "Currently on Row"=w1185) -> ("Table Out"=w1186:T6[], "noWaitCompletion"=w1182:timestamp, "remainingTime"=w1180:string)  [unwired: 1 out]
            n582 = Decrement(x=w1192) -> (x-1=w1194:i32)
            n583 = local write "remainingTime"(w1180) -> ()
            n584 = Equal To 0?(x=w1182) -> (x = 0?=w1181:bool)
            n585 = Index Array(array=w1186, index=w1194) -> (element=w1193:T6)
            n586 = case shown="False" w1181 {
              tunnel: w1182 -> [w1195 _]
              frame False {
                "PredictedEnd" <- w1195
              }
              frame True {
              }
            }
            n587 = Unbundle By Name(w1193) -> ("EstCompl"=w1191:string)
            n588 = call "Program_Active_Client.vi"("Mode"=enum16{"Program Active", "Traverse Level State"}."Traverse Level State", "Traverse level State"=Traverse_Level_State."Running") -> ()  [unwired: 1 in, 3 out]
          }
        }
        "Estimated Completion" <- w1155
        n589 = global write "Trav_pos_global.vi" "Estimated Completion time"(w1155) -> ()
      }
      frame "Pause Multi Run Program" {
        n590 = while {
          tunnel: "Pause" -> [w1212]
          tunnel: [w1215] -> w1207
          tunnel: w1206 -> [w1214]
          tunnel: w1204 -> [w1213]
          shift-right: [w1212] -> _
          shift-left: _ -> [w1211]
          stop <- TRUE stop-if-true
          n591 = case shown="False" w1212 {
            selector: w1212 -> [_ w1217]
            tunnel: [w1216 w1221] -> w1215
            tunnel: w1214 -> [w1216 w1219]
            tunnel: w1213 -> [_ w1220]
            tunnel: w1211 -> [_ w1218]
            frame False {
            }
            frame True {
              n592 = stacked-sequence {
                tunnel: w1219 -> [_ _ _ _ w1236]
                tunnel: [_ _ _ _ w1237] -> w1221
                tunnel: w1220 -> [w1223 _ _ _ _]
                tunnel: w1217 -> [_ _ _ w1232 _]
                tunnel: w1218 -> [_ _ _ w1231 _]
                frame #0 {
                  n593 = Quotient & Remainder(x=w1223, y=15) -> (x-y*floor(x/y)=w1222:i32)  [unwired: 1 out]
                  n594 = case shown="0" w1222 {
                    frame 0 {
                      n595 = Current VI's Path() -> (path=w1225:path)
                      n596 = call "Bring_to_front.vi"("path"=w1225) -> ()
                    }
                    frame 1, Default {
                    }
                  }
                }
                frame #1 {
                  n597 = global write "Trav_pos_global.vi" "Paused During Row?"(TRUE ("Paused During Row?")) -> ()
                  "Pause message" <- "Multi Run Program Paused!!!!" ("Pause message")
                }
                frame #2 {
                  n598 = property on="Pause message" class="Str"("Visible"=TRUE) -> ()  [unwired: 2 in, 2 out]
                  n599 = Wait Until Next ms Multiple(millisecond multiple=u32 1500) -> ()  [unwired: 1 out]
                }
                frame #3 {
                  n600 = Compound Arithmetic op=AND(w1232, invert w1231) -> (w1230:bool)
                  n601 = case shown="True" w1230 {
                    frame False {
                    }
                    frame True {
                      n602 = call "Program_Active_Client.vi"("Mode"=enum16{"Program Active", "Traverse Level State"}."Program Active", "Time till next contact (Sec)"=12000.0, "Traverse level State"=Traverse_Level_State."Running") -> ()  [unwired: 3 out]
                    }
                  }
                }
                frame #4 {
                  n603 = property on="Pause message" class="Str"("Visible"=FALSE) -> ()  [unwired: 2 in, 2 out]
                  n604 = Wait Until Next ms Multiple(millisecond multiple=u32 1500) -> ()  [unwired: 1 out]
                  n605 = Decrement(x=w1236) -> (x-1=w1237:T3)
                }
              }
            }
          }
        }
        n606 = call "Overhead_Factor.vi"("Mode"=Overhead."Read Current Overhead") -> ("Current Overhead Factor"=→"Overhead Factor":dbl)  [unwired: 3 in]
      }
      frame "Do Another Row?" {
        w1249 = Multi_Run_Status."Terminate Run" ("Status")
        n607 = global read "Preference_global.vi" "Server Comms"() -> (w1244:T27)
        n608 = case shown="\"Server Link Healthy\"" w1244 {
          tunnel: [w1259 TRUE] -> w1243
          frame "Server Link Healthy" {
            n609 = call "Get_Current_Scan_client.vi"("singleChannel"="EnFlo Lab:Emergency_Stop:Happy") -> ("Numerical Values"=w1262:dbl[])  [unwired: 1 in, 3 out]
            n610 = Index Array(array=w1262) -> (element=w1260:dbl)  [unwired: 1 in]
            n611 = Not A Number/Path/Refnum?(number/path/refnum=w1260) -> (NaN/Path/Refnum?=w1261:bool)
            n612 = case shown="True" w1261 {
              tunnel: w1260 -> [w1265 _]
              tunnel: [w1263 TRUE] -> w1259
              frame False {
                n613 = Greater?(x=w1265, y=0.5) -> (0:w1263:bool)
              }
              frame True {
              }
            }
          }
          frame "Do Not Link To Server" {
          }
        }
        n614 = case shown="False" "Stop after Repeats" {
          tunnel: w1245 -> [_ w1271]
          frame False {
            n615 = local read "Current Row"() -> (w1269:i32)
            n616 = Increment(x=w1269) -> (x+1=→"Last Row Run":i32)
          }
          frame True {
            n617 = Decrement(x=w1271) -> (x-1=w1270:i32)
            n618 = local write "Current Row"(w1270) -> ()
          }
        }
        n619 = case shown="False" "stop" {
          tunnel: [w1272 w1273] -> w1250
          tunnel: w1249 -> [_ w1273]
          frame False {
            n620 = local read "Status"() -> (w1272:T2)
          }
          frame True {
            n621 = local write "Status"(w1273) -> ()
          }
        }
        n622 = Not Equal?(x=w1249, y=w1250) -> (x != y?=w1248:bool)
        n623 = case shown="False" w1248 {
          tunnel: [w1274 w1278] -> w1241
          tunnel: w1253 -> [w1275 _]
          tunnel: w1250 -> [_ w1279]
          frame False {
            n624 = case shown="\"Check VI only\"" w1275 {
              tunnel: [Multi_Run_Case."Show jumped positions" ("Multi Run Case") Multi_Run_Case."Shut down source etc" ("Multi Run Case")] -> w1274
              frame "Check VI only" {
              }
              frame "Run VI" {
              }
            }
          }
          frame True {
            n625 = case shown="\"Jump To Fall Back\"" w1279 {
              tunnel: [Multi_Run_Case."Skip Blank Rows" ("Multi Run Case") Multi_Run_Case."Find Next Fall Back Row" ("Multi Run Case")] -> w1278
              frame "Continue", Default {
              }
              frame "Jump To Fall Back" {
              }
            }
          }
        }
        n626 = local read "Display Mode"() -> (w1240:T5)
        n627 = case shown="True" w1243 {
          tunnel: [Multi_Run_Case."Shut down source etc" ("Multi Run Case") w1257] -> w1242
          tunnel: w1241 -> [_ w1257]
          frame False {
            n628 = local write "Status"(Multi_Run_Status."Terminate Run" ("Status")) -> ()
          }
          frame True {
          }
        }
        n629 = global write "Route_mapping_global.vi" "Display Mode"(w1240) -> ()
      }
      frame "Find Next Fall Back Row" {
        n630 = local read "Current Row"() -> (w1288:i32)
        n631 = global write "Trav_pos_global.vi" "MultiRun Has Jumped?"(TRUE ("MultiRun Has Jumped?")) -> ()
        n632 = Increment(x=w1288) -> (x+1=w1292:i32)
        n633 = Greater?(x=w1291, y=w1292) -> (0:w1297:bool)
        n634 = Index Array(array=w1289, index=w1288) -> (element=w1286:T6)
        n635 = Unbundle By Name(w1286) -> ("Comments"=w1282:string, "Row Type Selector"=w1287:T8)
        n636 = Equal?(x=w1287, y=Multi_run_mode."Fall Back to this Row" ("Mode")) -> (x = y?=w1293:bool)
        n637 = case shown="True" w1297 {
          tunnel: [Multi_Run_Case."Skip Blank Rows" ("Multi Run Case") w1304] -> w1296
          tunnel: w1293 -> [_ w1300]
          tunnel: w1288 -> [_ w1301]
          frame False {
          }
          frame True {
            n638 = case shown="False" w1300 {
              tunnel: w1301 -> [w1306 _]
              frame False {
                n639 = Increment(x=w1306) -> (x+1=w1305:i32)
                n640 = local write "Current Row"(w1305) -> ()
              }
              frame True {
              }
            }
            n641 = Select(t=Multi_Run_Case."Skip Blank Rows" ("Multi Run Case"), s=w1300, f=Multi_Run_Case."Find Next Fall Back Row" ("Multi Run Case")) -> (s? t:f=w1304:T3)
          }
        }
        n642 = Concatenate Strings(w1282, " !!Program added comments Jumped") -> (w1284:string)
        n643 = Bundle By Name(cluster=w1286, "Comments"=w1284) -> (w1285:T6)
        n644 = Replace Array Subset(array=w1289, new element=w1285, index=w1288) -> ()  [unwired: 1 out]
      }
      frame "Shut down source etc" {
        w1312 = u32 1  # Time to hold source OFF (microseconds)
        w1313 = u32 0  # Time to hold source ON (microseconds)
        n645 = global read "Trav_pos_global.vi" "Default Gas Line Name"() -> (w1314:T25)
        n646 = global read "Extra_Commands_Global.vi" "Gas Line Name"() -> (w1310:string)
        n647 = for {
          tunnel: w1334 -> [w1360] mode=indexing
          tunnel: Multi_run_mode."Synchronize With:" ("Mode") -> [w1358]
          tunnel: [w1357] -> w1336 mode=indexing
          tunnel: w1310 -> [w1355]
          tunnel: [w1354] -> w1309 mode=indexing if=w1353
          n648 = Unbundle By Name(w1360) -> ("Extra Commands"=w1356:string, "Row Type Selector"=w1359:T8)
          n649 = Equal?(x=w1359, y=w1358) -> (x = y?=w1357:bool)
          n650 = call "Extra_Commands.vi"("String to Search"=w1356, "Command"=w1355) -> ("String Value"=w1354:string, "Command Found"=w1353:bool)  [unwired: 1 in, 3 out]
        }
        n651 = call "Set_Source.vi"("Source Establishment Time (s)"=0.0, "Source Status"=Client_Source_Status."Not Using", "Gas Line Name"=w1314, "Simulate/Run"=User_Specific_mode."Run VI") -> ()  [unwired: 1 in, 6 out]
        n652 = call "Program_Active_Client.vi"("Mode"=enum16{"Program Active", "Traverse Level State"}."Traverse Level State", "Traverse level State"=Traverse_Level_State."Complete") -> ()  [unwired: 1 in, 3 out]
        n653 = call "Overhead_Factor.vi"("Mode"=Overhead."Re Scale totals to 3 hrs") -> ()  [unwired: 3 in, 1 out]
        n654 = local read "Status"() -> (w1324:T2)
        n655 = global read "Meas_global.vi" "Start Time of experiment"() -> (w1332:dbl)
        n656 = Equal?(x=w1324, y=Multi_Run_Status."Terminate Run" ("Status")) -> (x = y?=w1322:bool)
        n657 = Or Array Elements(Boolean array=w1336) -> (logical OR=w1325:bool)
        n658 = call "Analyse_string_array.vi"("String array"=w1309) -> ("Unique strings"=w1308:string[])  [unwired: 1 in, 1 out]
        n659 = for {
          tunnel: w1308 -> [w1342] mode=indexing
          n660 = call "Gas line En-Type.vi"("Gas Line Name String"=w1342) -> ("Gas Line Name"=w1343:T25)  [unwired: 4 in]
          n661 = call "Set_Source.vi"("Source Establishment Time (s)"=0.0, "Source Status"=Client_Source_Status."Not Using", "Gas Line Name"=w1343, "Simulate/Run"=User_Specific_mode."Run VI") -> ()  [unwired: 1 in, 6 out]
        }
        n662 = Compound Arithmetic op=AND(w1325, invert w1322) -> (w1326:bool)
        n663 = Get Date/Time In Seconds() -> (seconds since 1Jan1904=w1317:timestamp)
        n664 = case shown="True" w1326 {
          frame False {
          }
          frame True {
            n665 = global read "Preference_global.vi" "Rig Setup"() -> (w1346:string)
            n666 = Concatenate Strings(w1346, ":Program:Sync") -> (w1348:string)
            n667 = Bundle By Name(cluster=T22 {"Channel Name"="", "New Value"=0.0, "!Auto_Off"=FALSE} ("Update Scan Value Cluster"), "Channel Name"=w1348, "New Value"=1000.0 ("Bundle Element")) -> (w1349:T22)
            n668 = Build Array(w1349) -> (w1351:T22[])
            n669 = call "Update_Current_Value_client.vi"("Update array in"=w1351) -> ()  [unwired: 1 in]
          }
        }
        n670 = To Double Precision Float(number=w1317) -> (double precision float=w1333:dbl)
        n671 = Subtract(x=w1333, y=w1332) -> (x-y=w1331:dbl)
        n672 = Greater?(x=w1331, y=1800.0) -> (0:w1328:bool)
        n673 = Not(x=w1328) -> (.not. x?=→"Non Starter":bool)
        n674 = Increment(x=w1320) -> (x+1=w1319:T3)
        n675 = Increment(x=w1319) -> (x+1=w1318:T3)
        n676 = call "Arduino_Timed_Release.vi"("Time to hold source ON (microseconds)"=w1313, "Time to hold source OFF (microseconds)"=w1312, "Number of cycles"=u16 1) -> ()  [unwired: 2 out]
        n677 = Select(t=w1320, s=w1328, f=w1318) -> (s? t:f=w1329:T3)
      }
      frame "Email results to users" {
        n678 = local read "Current Row"() -> (w1369:i32)
        n679 = Increment(x=w1369) -> (x+1=w1365:i32)
        n680 = global read "Trav_pos_global.vi" "MultiRun Has Jumped?"() -> (w1363:bool)
        n681 = Split 1D Array(array=w1366, index=w1365) -> (first subarray=w1373:T6[], second subarray=w1372:T6[])
        n682 = Array Size(array=w1372) -> (size(s)=w1374:i32)
        n683 = Greater Than 0?(x=w1374) -> (x > 0?=w1364:bool)
        n684 = Or(x=w1364, y=w1363) -> (x .or. y?=w1362:bool)
        n685 = case shown="True" w1362 {
          tunnel: ["" "Having completed only some of the requested rows." ("Message")] -> w1370
          frame False {
          }
          frame True {
          }
        }
        n686 = global read "Trav_pos_global.vi" "Results File Prefix"() -> (w1361:string)
        n687 = for {
          tunnel: w1373 -> [w1390] mode=indexing
          shift-right: [w1388] -> w1375
          shift-left: string[] [] -> [w1389]
          tunnel: w1361 -> [w1380]
          n688 = Unbundle By Name(w1390) -> ("Row Type Selector"=w1381:T8, "Filename"=w1387:path, "Comments"=w1386:string)
          n689 = Not Equal?(x=Multi_run_mode."Auto Calibrate" ("Row Type Selector"), y=w1381) -> (x != y?=w1383:bool)
          n690 = Empty String/Path?(string/path=w1387) -> (empty?=w1384:bool)
          n691 = Compound Arithmetic op=AND(w1383, invert w1384) -> (w1382:bool)
          n692 = case shown="True" w1382 {
            tunnel: w1389 -> [w1391 w1402]
            tunnel: [w1391 w1401] -> w1388
            tunnel: w1387 -> [_ w1399]
            tunnel: w1386 -> [_ w1400]
            tunnel: w1380 -> [_ w1395]
            frame False {
            }
            frame True {
              n693 = Strip Path(path=w1399) -> (name=w1394:string)  [unwired: 1 out]
              n694 = Match Pattern(string=w1400, regular expression=" !!Program added comments") -> (after substring=w1393:string)  [unwired: 4 out]
              n695 = Concatenate Strings(w1395, w1394, w1393) -> (w1392:string)
              n696 = Equal?(x=w1393, y=" Jumped") -> (x = y?=w1396:bool)
              n697 = case shown="True" w1396 {
                tunnel: w1402 -> [w1405 w1406]
                tunnel: [w1404 w1406] -> w1401
                tunnel: w1392 -> [w1403 _]
                frame False {
                  n698 = Build Array (concatenate)(w1405, w1403) -> (w1404:string[])
                }
                frame True {
                }
              }
            }
          }
        }
        n699 = call "End_of_run_messages.vi"("Message"=w1370, "Subject"="Multi Run Ended", "Attachments"=w1375) -> ()  [unwired: 1 in]
      }
      frame "Save run efficiency" {
        n700 = global read "Preference_global.vi" "Preferences for computer"() -> (w1412:path)
        n701 = call "Overhead_Factor.vi"("Mode"=Overhead."Read Current Overhead") -> ("Current Overhead Factor"=w1410:dbl)  [unwired: 3 in]
        n702 = call <vilib>:"Open Config Data.vi"("configuration file path"=w1412) -> ("refnum"=w1408:T28)  [unwired: 8 in, 2 out]
        n703 = call-poly <vilib>:"Write Key.vi"("section"="PreferencePanel", "value"=w1410, "key"="Current Overhead Factor", "refnum"=w1408) -> ("refnum out"=w1407:T28)  [unwired: 5 in, 2 out]
        n704 = call <vilib>:"Close Config Data.vi"("refnum"=w1407) -> ()  [unwired: 9 in, 2 out]
      }
      frame "Remove Skipped Commands" {
        n705 = for {
          tunnel: w1425 -> [w1433] mode=indexing
          tunnel: [w1432] -> w1424 mode=indexing
          n706 = Unbundle By Name(w1433) -> ("Comments"=w1431:string)
          n707 = Match Pattern(string=w1431, regular expression=" !!Program added comments") -> (before substring=w1430:string)  [unwired: 4 out]
          n708 = Bundle By Name(cluster=w1433, "Comments"=w1430) -> (w1432:T6)
        }
        n709 = Current VI's Path() -> (path=w1419:path)
        n710 = Open VI Reference(vi path=w1419) -> (vi reference=w1420:refnum<vi>, error out=w1421:errorcluster)  [unwired: 1 in, 4 out]
        n711 = property class="VI"(reference=w1420, error in=w1421, "Front Panel Window:Is Frontmost"=TRUE) -> (reference out=w1422:refnum<vi>, error out=w1423:errorcluster)
        n712 = Close Reference(reference=w1422, error in (no error)=w1423) -> ()  [unwired: 1 out]
      }
      frame "Show jumped positions" {
        n713 = local read "Command filename"() -> (w1442:path)
        n714 = call "MultiRun Status.vi"() -> ("Table Control"=w1436:string[][])  [unwired: 1 in]
        n715 = Strip Path(path=w1442) -> (stripped path=w1438:path)  [unwired: 1 out]
        n716 = Array To Spreadsheet String(array=w1436, 3:"%s" ("format string")) -> (spreadsheet string=w1434:string)  [unwired: 1 out]
        n717 = Build Path(base path=w1438, name or relative path="Multi_Run_Status_Report.xls" ("format string")) -> (appended path=w1440:path)
        n718 = call "Create_directory_path.vi"("Dialog Box"=FALSE, "Path name"=w1440) -> ("Path name Out"=w1435:path)  [unwired: 1 in, 1 out]
        n719 = call "Write Characters with check.vi"("String to Write"=w1434, "file (use dialog)"=w1435) -> ()  [unwired: 2 in, 1 out]
      }
      frame "Save Setup to File" {
        w1463 = FALSE  # Start of Multi Run Prog
        n720 = local read "Command filename"() -> (w1447:path)
        n721 = local read "Status"() -> (w1458:T2)
        n722 = local read "Stop after Repeats"() -> (w1461:bool)
        n723 = local read "Last Row Run"() -> (w1451:i32)
        n724 = local read "stop"() -> (w1462:bool)
        n725 = local read "Non Starter"() -> (w1449:bool)
        n726 = Less?(x=w1458, y=Multi_Run_Status."Jump to Next Point" ("Status")) -> (x < y?=w1457:bool)
        n727 = Less?(x=w1456, y=T9."Run Multi Run Prog") -> (x < y?=w1450:bool)
        n728 = Decrement(x=w1451) -> (x-1=w1454:i32)
        n729 = Equal?(x=w1452, y=w1451) -> (x = y?=w1470:bool)
        n730 = Equal To 0?(x=w1451) -> (x = 0?=w1469:bool)
        n731 = Compound Arithmetic op=OR(w1461, w1462, w1457) -> (w1460:bool)
        n732 = Select(t=w1451, s=w1460, f=w1454) -> (s? t:f=w1464:i32)
        n733 = Compound Arithmetic op=OR(w1470, w1469, w1450, w1449) -> (w1471:bool)
        n734 = Split 1D Array(array=w1475, index=w1464) -> (second subarray=w1478:T6[])  [unwired: 1 out]
        n735 = local read "Work in Tunnel Coordinates?"() -> (w1453:T1)
        n736 = Path To String(path=w1447) -> (string=w1468:string)
        n737 = local read "Fast Plotting?"() -> (w1448:bool)
        n738 = case shown="False" w1471 {
          tunnel: w1447 -> [w1487 w1521]
          tunnel: [w1486 w1521] -> w1479
          tunnel: w1478 -> [w1484 _]
          tunnel: [w1483 w1522] -> w1477
          tunnel: w1475 -> [w1485 w1522]
          tunnel: w1453 -> [w1482 _]
          tunnel: w1448 -> [w1481 _]
          frame False {
            n739 = stacked-sequence {
              tunnel: w1487 -> [w1490 w1500 _]
              tunnel: [_ w1493 _] -> w1486
              tunnel: w1485 -> [w1492 _ w1505]
              tunnel: w1484 -> [_ _ w1503]
              tunnel: [_ _ w1502] -> w1483
              tunnel: w1482 -> [w1491 _ _]
              tunnel: w1481 -> [w1488 _ _]
              frame #0 {
                n740 = global write "Trav_pos_global.vi" "Sync to server now"(TRUE) -> ()
                n741 = call "Save_Trav_setup.vi"("Work in Tunnel Coordinates?"=w1491, "Trav Table"=w1492, "Fast Plotting?"=w1488, "Setup filename"=w1490) -> ()  [unwired: 1 in, 1 out]
              }
              frame #1 {
                n742 = Strip Path(path=w1500) -> (stripped path=w1501:path, name=w1499:string)
                n743 = call "Add_filename_suffix.vi"("Filename"=w1499) -> ("Original Suffix"=w1496:string, "Base name"=w1498:string)  [unwired: 1 in, 2 out]
                n744 = Concatenate Strings(w1498, "_Rem", w1496) -> (w1495:string)
                n745 = Build Path(base path=w1501, name or relative path=w1495) -> (appended path=w1494:path)
                n746 = call "Find_Unique_Filename.vi"("Path In"=w1494) -> ("Unique Path Out"=w1493:path)  [unwired: 1 in, 1 out]
              }
              frame #2 {
                n747 = global read "Extra_Commands_Global.vi" "Minutes Before Repeating Row"() -> (w1506:string)
                n748 = Index Array(array=w1505, index=0) -> (element=w1508:T6)
                n749 = Initialize Array(w1508, 0 ("dimension size")) -> (w1507:T6[])
                n750 = for {
                  shift-right: [w1511] -> w1504
                  shift-left: w1507 -> [w1513]
                  tunnel: w1506 -> [w1515]
                  tunnel: w1505 -> [w1512] mode=indexing
                  n751 = Unbundle By Name(w1512) -> ("Extra Commands"=w1514:string)
                  n752 = call "Extra_Commands.vi"("String to Search"=w1514, "Command"=w1515) -> ("Command Found"=w1516:bool)  [unwired: 1 in, 4 out]
                  n753 = case shown="True" w1516 {
                    tunnel: w1513 -> [w1517 w1520]
                    tunnel: w1512 -> [_ w1519]
                    tunnel: [w1517 w1518] -> w1511
                    frame False {
                    }
                    frame True {
                      n754 = Build Array (concatenate)(w1520, w1519) -> (w1518:T6[])
                    }
                  }
                }
                n755 = Build Array (concatenate)(w1504, w1503) -> (w1502:T6[])
              }
            }
          }
          frame True {
          }
        }
        n756 = Concatenate Strings("Multi run Prog Ended having the setup filename of :" ("Message"), w1468) -> (w1467:string)
        n757 = call "Log_Current_row_to_Execute.vi"("Simulate/Run"=w1466, "Message"=w1467, "Start of Multi Run Prog"=w1463) -> ()  [unwired: 2 in, 5 out]
        n758 = call "Save_Trav_setup.vi"("Work in Tunnel Coordinates?"=w1453, "Trav Table"=w1477, "Fast Plotting?"=w1448, "Setup filename"=w1479) -> ("Trav Table Out"=w1476:T6[])  [unwired: 1 in]
        n759 = Select(t=w1476, s=w1471, f=w1475) -> (s? t:f=w1474:T6[])
      }
      frame "End" {
        n760 = stacked-sequence {
          frame #0 {
            w1528 = ""
            w1529 = path ""
            w1530 = 0 ("No. of pts.")
            w1527 = nan
            n761 = global write "Trav_pos_global.vi" "Top level setup filename"(w1529) -> ()
            n762 = global read "Trav_pos_global.vi" "Current Row"() -> (w1534:T6)
            n763 = Bundle By Name(cluster=w1534, "Start X"=w1527, "Start Y"=w1527, "Start Z"=w1527, "End X"=w1527, "End Y"=w1527, "End Z"=w1527, "nPoints"=w1530, "Spacing"=Spacing."Linear", "Filename"=w1529, "Tunnel Speed"=w1527, "Averaging time (mins)"=w1527, "Extra Commands"=w1528, "Specific Arguments"=w1528, "Carrier_1 Q (l/min)"=w1527, "Trace Gas Concentration (%)"=w1527, "Carrier_2 Q (l/min)"=w1527, "Comments"=w1528, "Row No"=w1530, "Row Type Selector"=Multi_run_mode."Blank Row", "EstCompl"=w1528, "Meas Setup File"=w1528, "Row Duration (mins)"=w1527, "nValidPoints"=w1530) -> (w1533:T6)
            n764 = global write "Trav_pos_global.vi" "Current Row"(w1533) -> ()
          }
          frame #1 {
            n765 = local read "Command filename"() -> (w1544:path)
            n766 = global write "Preference_global.vi" "Send Emails?"(FALSE ("Send Emails?")) -> ()
            n767 = call "LDA_Mirror_Setup.vi"("Simulate/Run"=User_Specific_mode."Run VI") -> ()  [unwired: 3 in, 1 out]
            n768 = global write "Trav_pos_global.vi" "Estimated Completion time"("") -> ()
            n769 = call "Current_Filepath.vi"("Short_Name"="Cmd" ("Data Type"), "Filename in"=w1544, "Data Type"="Commands") -> ()  [unwired: 1 in, 2 out]
            n770 = local read "Fast Plotting?"() -> (w1538:bool)
            n771 = global write "Trav_pos_global.vi" "Measurement setup files"(string[] [] ("Measurement setup files")) -> ()
            n772 = case shown="True" w1538 {
              frame False {
              }
              frame True {
                n773 = call "Shut_down_all_Axis.vi"() -> ()  [unwired: 1 in, 1 out]
              }
            }
            n774 = global write "Trav_pos_global.vi" "Fast Plotting?"(FALSE ("Fast Plotting?")) -> ()
            n775 = global write "Trav_pos_global.vi" "Meas Setup Number"(0 ("Meas Setup Number")) -> ()
            n776 = Build Array(u32 0) -> (w1536:u32[])
            n777 = property on="Table" class="Arr (strict)"("Index Values"=w1536) -> ()  [unwired: 2 in, 2 out]
          }
          frame #2 {
            n778 = Current VI's Path() -> (path=w1547:path)
            n779 = call "Bring_to_front.vi"("path"=w1547) -> ()
          }
        }
      }
    }
    n780 = case shown="True" w15 {
      tunnel: w13 -> [_ w21]
      frame False {
      }
      frame True {
        n781 = local write "Table"(w21) -> ()
      }
    }
    "Case" <- w17
  }
